vi "Module - Page Execute.vi"(11 "Stop":bool) -> ()   [LabVIEW 2020]
uses:
  Control/Setup - Sequence Data.ctl
  Control/Setup - Sequence Data Label.ctl
  Control/Page - Execute State.ctl
  <vilib>/Utility/NIReport.llb/NI_report.lvclass
  Control/Data to Execute.ctl
  Control/Transaction Info.ctl
  Control/Product Info.ctl
  Control/Acceptance Criteria Info.ctl
  Control/Execution Info.ctl
  Control/Results Info.ctl
  Control/Execute - Index of Elapse time.ctl
  Control/State - eFGV.ctl
  Control/Section.ctl
  <vilib>/Utility/miscctls.llb/LVPointDoubleTypeDef.ctl
  Control/State - FGV.ctl
  <vilib>/Utility/NIReport.llb/Report Type.ctl
  <vilib>/Utility/file.llb/Write Delimited Spreadsheet (string).vi
  <userlib>/_OpenG.lib/comparison/comparison.llb/Boolean Changed__ogtk.vi
  <vilib>/Utility/NIReport.llb/Append Report Text (str wrap).vi
  <vilib>/Utility/NIReport.llb/NI_ReportGenerationCore.lvlib
panel:
  out "SequenceNoFolder":string
  out "Test Status Ind":string
  out "Hold Time Remainder":dbl
  in  "TARE":bool caption="1"
  in  "End Mark":bool caption="1"
  in  "Test Type":string(combo)
  in  "Execute Tab":enum32{"Test", "Info", "Misc."}(tab)
  out "Holding Started":bool
  in  "Chart No":string
  out "Overall Status":bool
  in  "Table Reading":i32(listbox)
  out "% Test Completed":dbl format="%.1f %"
  out "%Pressure Stabilized":dbl caption="% Pressure Stabilized" format="%.1f %"
  out "Holding Pressure Drop (Psi)":dbl
  out "Low Pressure":bool
  in  "Pause/Resume":bool
  in  "Execute View":string="View"
  in  "Execute Reading":string="Reading"
  in  "Execute Key Value":string="Key Value" caption="Info"
  in  "Execute Info":string="Info" caption="Info"
  out "Blow Down  Test":bool
  out "Hold Time (hh:mm)":string
  out "Test Pressure":i32 format="%.0f psi"
  in  "tab - View Data":T1(tab)
  in  "Start Marker":u32(colorbox)=16860
  in  "Plot Colour":u32(colorbox)=16711680
  in  "Stop Marker":u32(colorbox)=1441830
  in  "Grid Colour":u32(colorbox)=35170
  out "Polar Plot":picture
  out "Linear Graph":cluster{"Time ,x":dbl[], "Magnitude ,y":sgl[]}(graph)
  in  "Statistic":i32(listbox)
  out "Key Value Remain Hold Time":string="00:00:00" caption="Holding Time"
  out "Key Value Recording Duration":string="00:00:00" caption="Recording Duration"
  out "Key Value Current Pressure (psi)":sgl caption="Current Pressure (psi)" format="%.1f psi"
  in  "Run Test":bool caption="1"
  out "Remain Hold Time":string="00:00:00"
  out "Holding Pressure (psi)":dbl
  out "Current Pressure (psi)":sgl format="%.1f"
  in  "Clear Mark":bool caption="1"
  in  "Start Mark":bool caption="1"
  in  "Finish":bool caption="1"
  out "Start Holding Datetime":string
  out "End Holding Datetime":string
  out "Recorded Holding Time":string
  out "Start Holding Pressure (psi)":string
  out "End Holding Pressure (psi)":string
  out "Different in Holding Pressure,psi(%)":string
  out "Permitted Holding Pressure Drop, psi%":string
  out "Recording Duration":string="00:00:00"
  in  "View":string(combo)
  out "Test Sequence":string
  out "Seq.No":string
  out "Variance":string
  out "Transaction Number":u16
  out "Test Requirement":string
  out "Test Media":string
  out "Notes":string
  out "PSL":string
  in  "Test System Description":string caption="Test System"
  out "Rework":bool caption="Rework?"
  out "Ref Order No.":dbl caption="Ref. Order No."
  out "NCR No.":string
  in  "Header multi-test 3":T2={"Seq.SelectRun 4"="Select", "Seq.Done"="Status", "Seq.No"="Run?", "Seq.No 2"="Test Sequence", "Seq.No 3"="No.", "Seq.No 4"="Test Req. ID", "Seq.No 5"="Test Requirement", "Seq.No 6"="Variance", "Seq.No 7"="Test Procedure", "Seq.No 8"="Section", "Seq.No 9"="Test Bunker", "Seq.No 10"="Test Media", "Seq.No 11"="Test Pressure (psi)", "Seq.No 12"="Cycle", "Seq.No 13"="Holding time (hh:mm)", "Seq.No 14"="Chart Scale", "Seq.No 15"="Blowdown? (y/n)", "Seq.No 16"="Actuator Pressure (psi)", "Seq.No 17"="Max. Blowdown Pressure (psi)"}
  out "Sequence List":T3[](array[typedef])
  in  "Label.Test":string="Test" caption="Test"
  out "Test Category list":string="SUT 9, Hydro"
  in  "Test System":string
  in  "Test Category":string
  out "Material Description":string caption="Material List"
  out "Material":string
  out "Project":string
  out "Customer Description":string caption="Customer List"
  in  "Test System Name":string
  in  "Procedure No./Ref.":string caption="X-Document No./Ref."
  out "Working Pressure":string
  in  "Test System":string
  out "Rev.":string
  out "Product Category":string
  out "BOM Rev.":dbl
  out "Sale Order":string caption="Sales Order"
  out "Customer":string
  out "NCR":string
  out "Order Number":string
  out "Quantity":u16=1 min=1 step=1
  out "Auto Stop Test":bool caption="Automatic Stop Test after Hold Time Countdown"
  out "Auto Set Marker":bool caption="Automatic set start marker upon pressure stabilized"
  in  "Header.Tool":T4={"Type "="Type", "Id"=" ID", "Description"="Description", "Serial No"="Serial No"} caption="Header Tool"
  out "Table.Tool":i32(listbox) caption="Detail Sensor"
  out "Table.Sensor":i32(listbox) caption="Detail Sensor"
  in  "Header.Sensor":T5={"Type "="Type", "Id"=" ID", "Description"="Description", "Serial No"="Serial No", "LP"="LP"} caption="Header Detail Sensor"
  in  "Label.Result":string="Result" caption="Result"
  out "Output Set Company":string
  out "ListBox.Output Set":string caption="Output Set"
  in  "Label.Production Order Details":string="Production Order Details" caption="Production Order Details"
  out "Indicator.Sub Operation":string caption="Sub Operation"
  out "Indicator.Confirmation No":u32 caption="Confirmation No"
  out "Indicator.Operation":string caption="Operation"
  out "Indicator.Sequence No":u16 caption="Sequence No"
  out "Indicator.Order Number":u32 caption="Order Number"
  in  "Label.Tools":string="Tools" caption="Tools"
  in  "Label.Sensor":string="Sensor" caption="Sensor"
  in  "Label.Additional Procedures No./Ref.":string="Additional Procedures No./Ref." caption="Additional Procedures No./Ref."
  out "Table.Procedure No./Ref.":i32(listbox)
  out "Acceptance Criteria":string="Acceptance Criteria"
  out "% Permitted Holding Pressure":string="% per hour (vs. start holding pressure)"
  out "% Test Pressure":string=" % on top of the test pressure"
  out "Permitted Holding Pressure Drop":dbl
  out "Max Start Holding Pressure":dbl caption="Maximum Start Of Holding Pressure"
  # "EXECUTE"
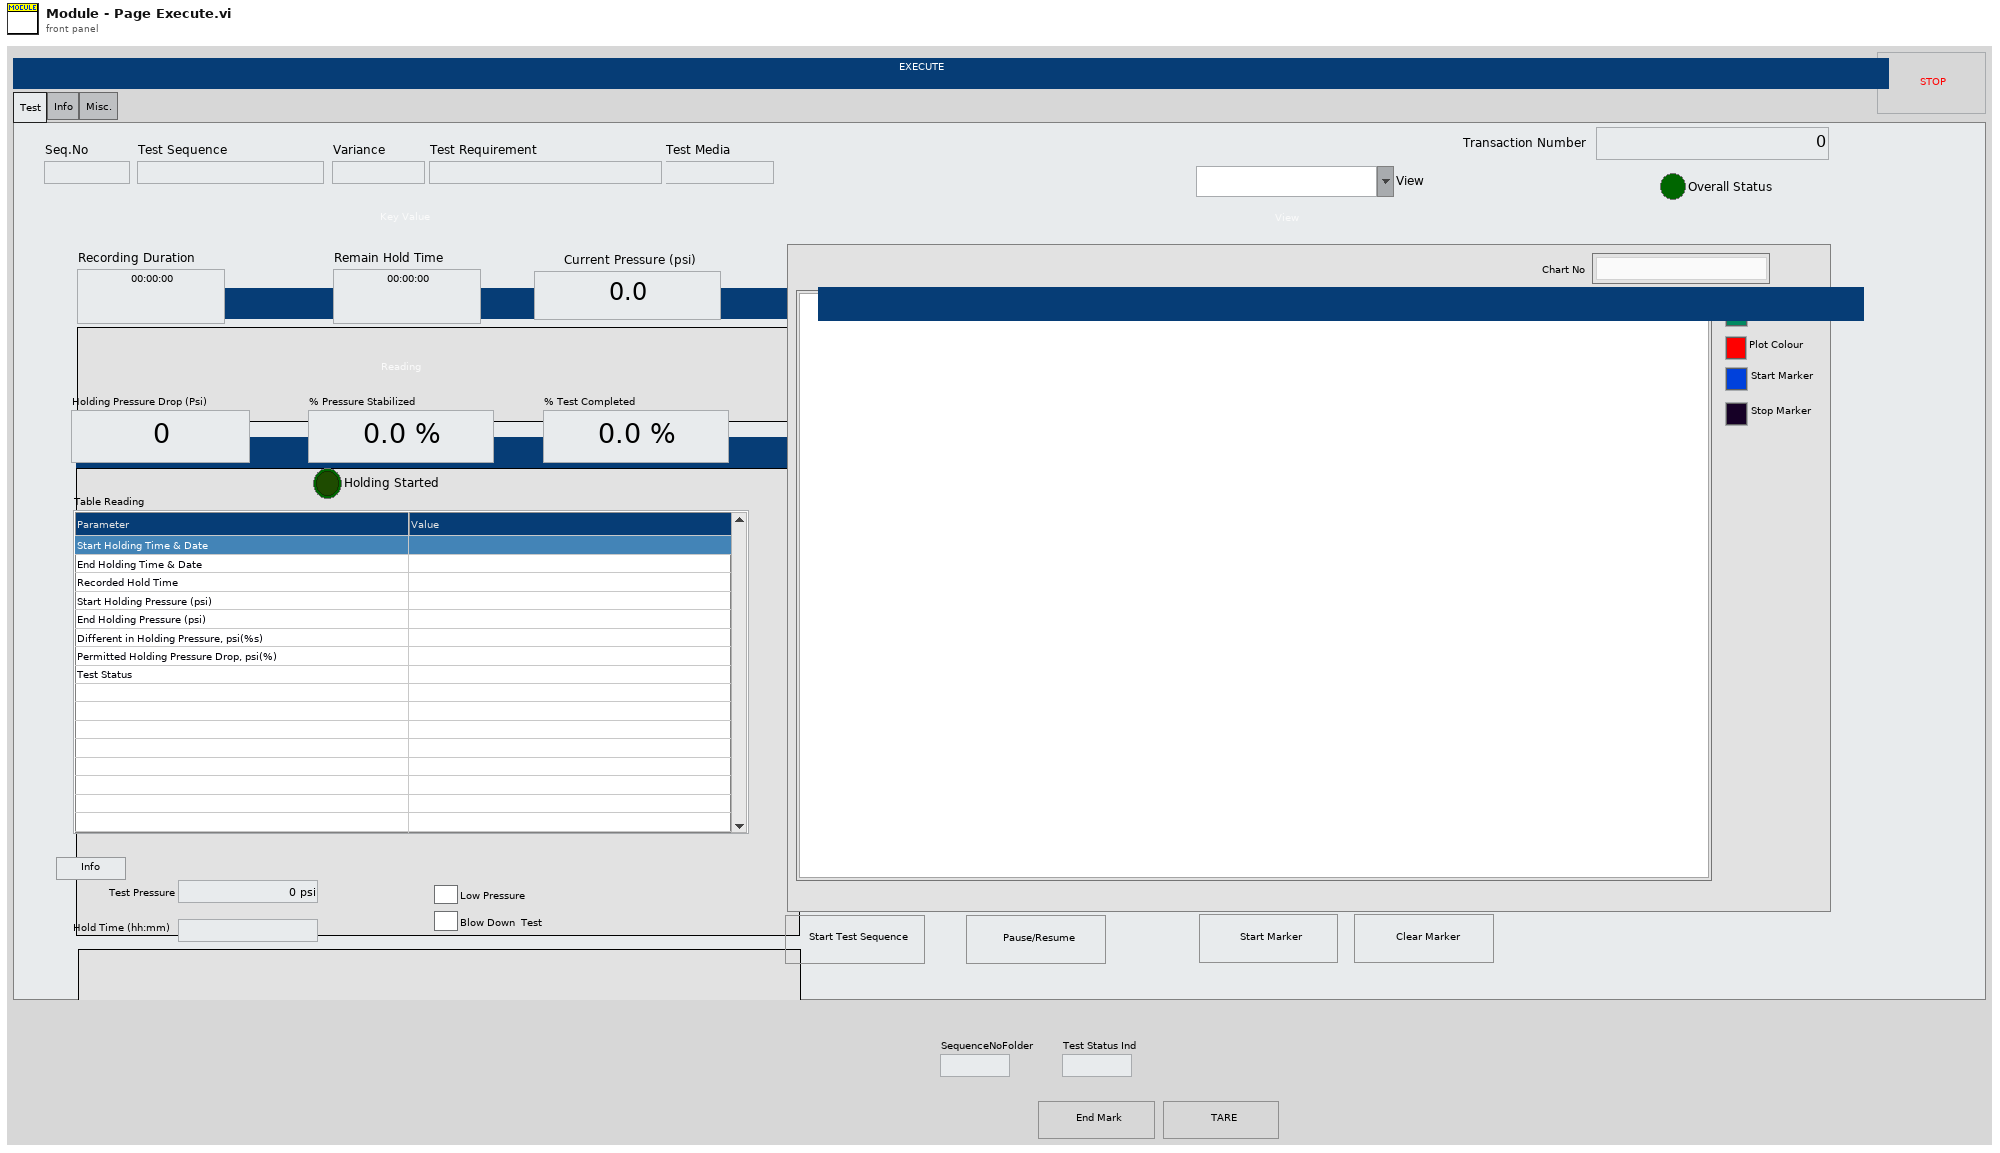
[diagram p1: front panel]
types:
  T1 = enum32{"Polar Plot", "Linear", "Statistic", "Key Value"}
  T2 = typedef "Setup - Sequence Data Label.ctl" = cluster{"Seq.SelectRun 4":string, "Seq.Done":string, "Seq.No":string, "Seq.No 2":string, "Seq.No 3":string, "Seq.No 4":string, "Seq.No 5":string, "Seq.No 6":string, "Seq.No 7":string, "Seq.No 8":string, "Seq.No 9":string, "Seq.No 10":string, "Seq.No 11":string, "Seq.No 12":string, "Seq.No 13":string, "Seq.No 14":string, "Seq.No 15":string, "Seq.No 16":string, "Seq.No 17":string}
  T3 = typedef "Setup - Sequence Data.ctl" = cluster{"Seq.Select":bool, "Seq.Status":u32, "Seq.Run":bool, "Seq.TestSequence":string, "Seq.No":string, "Seq.ReqID":string, "Seq.TestReq":string, "Seq.Variance":string, "Seq.TestProcedure":string, "Seq.Section":string, "Seq.TestBunker":string, "Seq.TestMedia":string, "Seq.TestPressure":string, "Seq.Cycle":string, "Seq.HoldingTime":string, "Seq.ChartScale":string, "Seq.BDIndicator":string, "Seq.ActuatorPressure":string, "Seq.MaxBDPressure":string}
  T4 = cluster{"Type ":string, "Id":string, "Description":string, "Serial No":string}
  T5 = cluster{"Type ":string, "Id":string, "Description":string, "Serial No":string, "LP":string}
  T6 = typedef "Execute - Index of Elapse time.ctl" = enum16{"Elapse Gap Data", "Holding Time", "Recording Duration"}
  T7 = typedef "Data to Execute.ctl" = cluster{"Transaction Info":T8, "Product Info":T9, "Misc - Additional Refs":string[][], "Misc - Sensors":string[][], "Misc - Tools":string[][], "Acceptance Criteria Info":T10, "Execution Info":T11, "Results Info":T12, "Notes":string}
  T8 = typedef "Transaction Info.ctl" = cluster{"Transaction Number":u32, "Order Number":u32, "Quantity":u16, "Customer":u32, "Customer Description":string, "Project":string, "Sales Order":u32, "Material":u32, "Material Description":string, "Rework":bool, "NCR No.":string, "Ref Order No.":dbl, "Item No.":u32, "BOM Rev.":dbl}
  T9 = typedef "Product Info.ctl" = cluster{"Product Category":string, "Procedure No./Ref.":string, "Test System":string, "Test System Description":string, "Working Pressure":string, "Pressure Unit":string, "Rev.":string, "PSL":string}
  T10 = typedef "Acceptance Criteria Info.ctl" = cluster{"Max Start Hold Pressure":dbl, "Enum.Max Start Hold Pressure":enum16{"%", "psi"}, "Permitted Hold Pressure Drop":dbl, "Enum.Permitted Hold Pressure Drop":enum16{"%", "psi"}}
  T11 = typedef "Execution Info.ctl" = cluster{"Auto Set Marker":bool, "Auto Stop Test":bool}
  T12 = typedef "Results Info.ctl" = cluster{"ListBox.Output Set":string, "Output Set Description":string}
  T13 = cluster{"T_Out":i32, "Point Phase":dbl[], "polar attributes":cluster{"maximum":dbl, "minimum":dbl, "clip to min":bool, "log?(F)":bool, "grid color":u32, "plot color":u32, "fmt and prec":cluster{"format":enum8{"Decimal", "Scientific", "Engineering", "Binary", "Octal", "Hex"}, "precision":u8}, "visible section":u16}, "Current Pressure":sgl, "Counter Time":dbl, "marking plot colour":u32, "Active Cursor":u32, "Event AI Data":sgl[], "Run Test":bool, "Config":cluster{"Holding Pressure":dbl, "Set Polar Time":dbl}, "Array of Elapse Time":timestamp[], "Remaining Holding Time":dbl, "Max Pressure":sgl, "Start Mark":bool, "Plot length (min)":dbl, "Plot length scale":dbl, "Magnitude ,y":sgl[], "Time ,x":dbl[], "Result Elapse":dbl[], "Phase":dbl[], "data array [mag, phase (deg)]":cluster{"magnitude":dbl, "phase":dbl}[], "Max Phase":dbl, "Plot and scale":cluster{"Size Linear plot":u16, "Size point plot":u16, "Plot Scale":dbl}, "Start Holding Pressure (psi)":dbl, "End Holding Pressure (psi)":dbl, "Marking Data":cluster{"magnitude 2":dbl, "phase":dbl}[], "Display Polar Scale":cluster{"Time Scale Label":string, "Max Scale label":string}, "report out":refnum<class "NI_report.lvclass">, "axis labels":string[], "Polar Picture":picture, "Event Ref":refnum<event-registration>, "Data to Execute":T7, "Sequence Data":T3[], "Holding Starter?":bool, "%Pressure Stabilized":dbl, "Target Holding Time":dbl, "Datalog path":path, "AI Offset":sgl[], "Sequence Number":i32, "Current Sequence":T3, "All Sequence Done":bool, "Sequence Started":bool}
  T14 = typedef "Page - Execute State.ctl" = enum16{"Init", "Register Event", "Read Config File", "Idle", "Start Marking", "Clear Mark", "Init Test Param", "Init File and Folder", "Get Current Sequence", "Cal Elapse Time", "Display Data", "Check Start Holding", "Polar attributes", "Insert Acc Data", "Convert Time To Phase", "Get Plot length", "Polar linear Plot", "Polar Point", "Plot linear Graph", "Update Table Data", "Display Holding Time", "Display Result Test", "Display Label", "Finish Test", "Setup Cop", "Merge Picture", "Save  Data", "Get Next Sequence", "Create Report", "Fillup Report", "Process", "Update Info - Transaction", "Update Info - Product", "Update Info - Additional Refs", "Update Info - Sensors", "Update Info - Tools", "Update Info - Acceptance Criteria", "Update Info - Execution", "Update Info - Results", "Update Info - Notes", "Close"}
  T15 = typedef "Section.ctl" = enum16{"Software Setup", "Config", "Setup", "Network Stream", "MQTT Client", "Setting", "Sample Interval", "Calibration", "Pre-Ranging", "Overrun", "Static", "Filter", "Properties", "Alarm", "Device", "Logging"}
  T16 = typedef "LVPointDoubleTypeDef.ctl" = cluster{"X":dbl, "Y":dbl}
  T17 = typedef "State - FGV.ctl" = enum16{"Write", "Read"}
  T18 = enum8{"Decimal", "Scientific", "Engineering", "Binary", "Octal", "Hex"}
  T19 = cluster{"polar attributes":cluster{"maximum":dbl, "minimum":dbl, "clip to min":bool, "log?(F)":bool, "grid color":u32, "plot color":u32, "fmt and prec":cluster{"format":enum8{"Decimal", "Scientific", "Engineering", "Binary", "Octal", "Hex"}, "precision":u8}, "visible section":u16}, "data array [mag, phase (deg)]":cluster{"magnitude":dbl, "phase":dbl}[], "font":cluster{"desired font(Application) ":enum16{"User-specified Font", "Application Font", "System Font", "Dialog Font"}, "[user-specified font] ":cluster{"Font Name:":string, "Size":i16, "Strikeout?":bool, "Italic?":bool, "Underline?":bool, "Outline?":bool, "Shadow?":bool, "Bold?":bool}}, "Scale Polar plot":dbl, "Size":u16}
  T20 = cluster{"Execute Data":string[], "Sequence no":string}
  T21 = typedef "State - eFGV.ctl" = enum16{"Init", "Read", "Write", "Exit"}
  T22 = typedef "NI_ReportGenerationCore.lvlib/Report Type.ctl" = enum16{"HTML", "Word", "Excel"}
  T23 = cluster{"position (excel)":cluster{"row":i32, "column":i32}, "name (excel)":string, "bookmark (word)":string}
  T24 = cluster{"Time Scale Label":string, "Max Scale label":string}
  T25 = cluster{"Size Linear plot":u16, "Size point plot":u16, "Plot Scale":dbl}
  T26 = cluster{"maximum":dbl, "minimum":dbl, "clip to min":bool, "log?(F)":bool, "grid color":u32, "plot color":u32, "fmt and prec":cluster{"format":enum8{"Decimal", "Scientific", "Engineering", "Binary", "Octal", "Hex"}, "precision":u8}, "visible section":u16}
  T27 = typedef "LVBoundsTypeDef.ctl" = cluster{"Width":u32, "Height":u32}
  T28 = typedef "imagedata.ctl" = cluster{"image type":i32, "image depth":i32, "image":u8[], "mask":u8[], "colors":u32[], "Rectangle":cluster{"left":i16, "top":i16, "right":i16, "bottom":i16}}
  T29 = enum32{"invalid app kind", "Development System", "Run Time System", "Student Edition", "Embedded LabVIEW", "Evaluation", "Custom"}
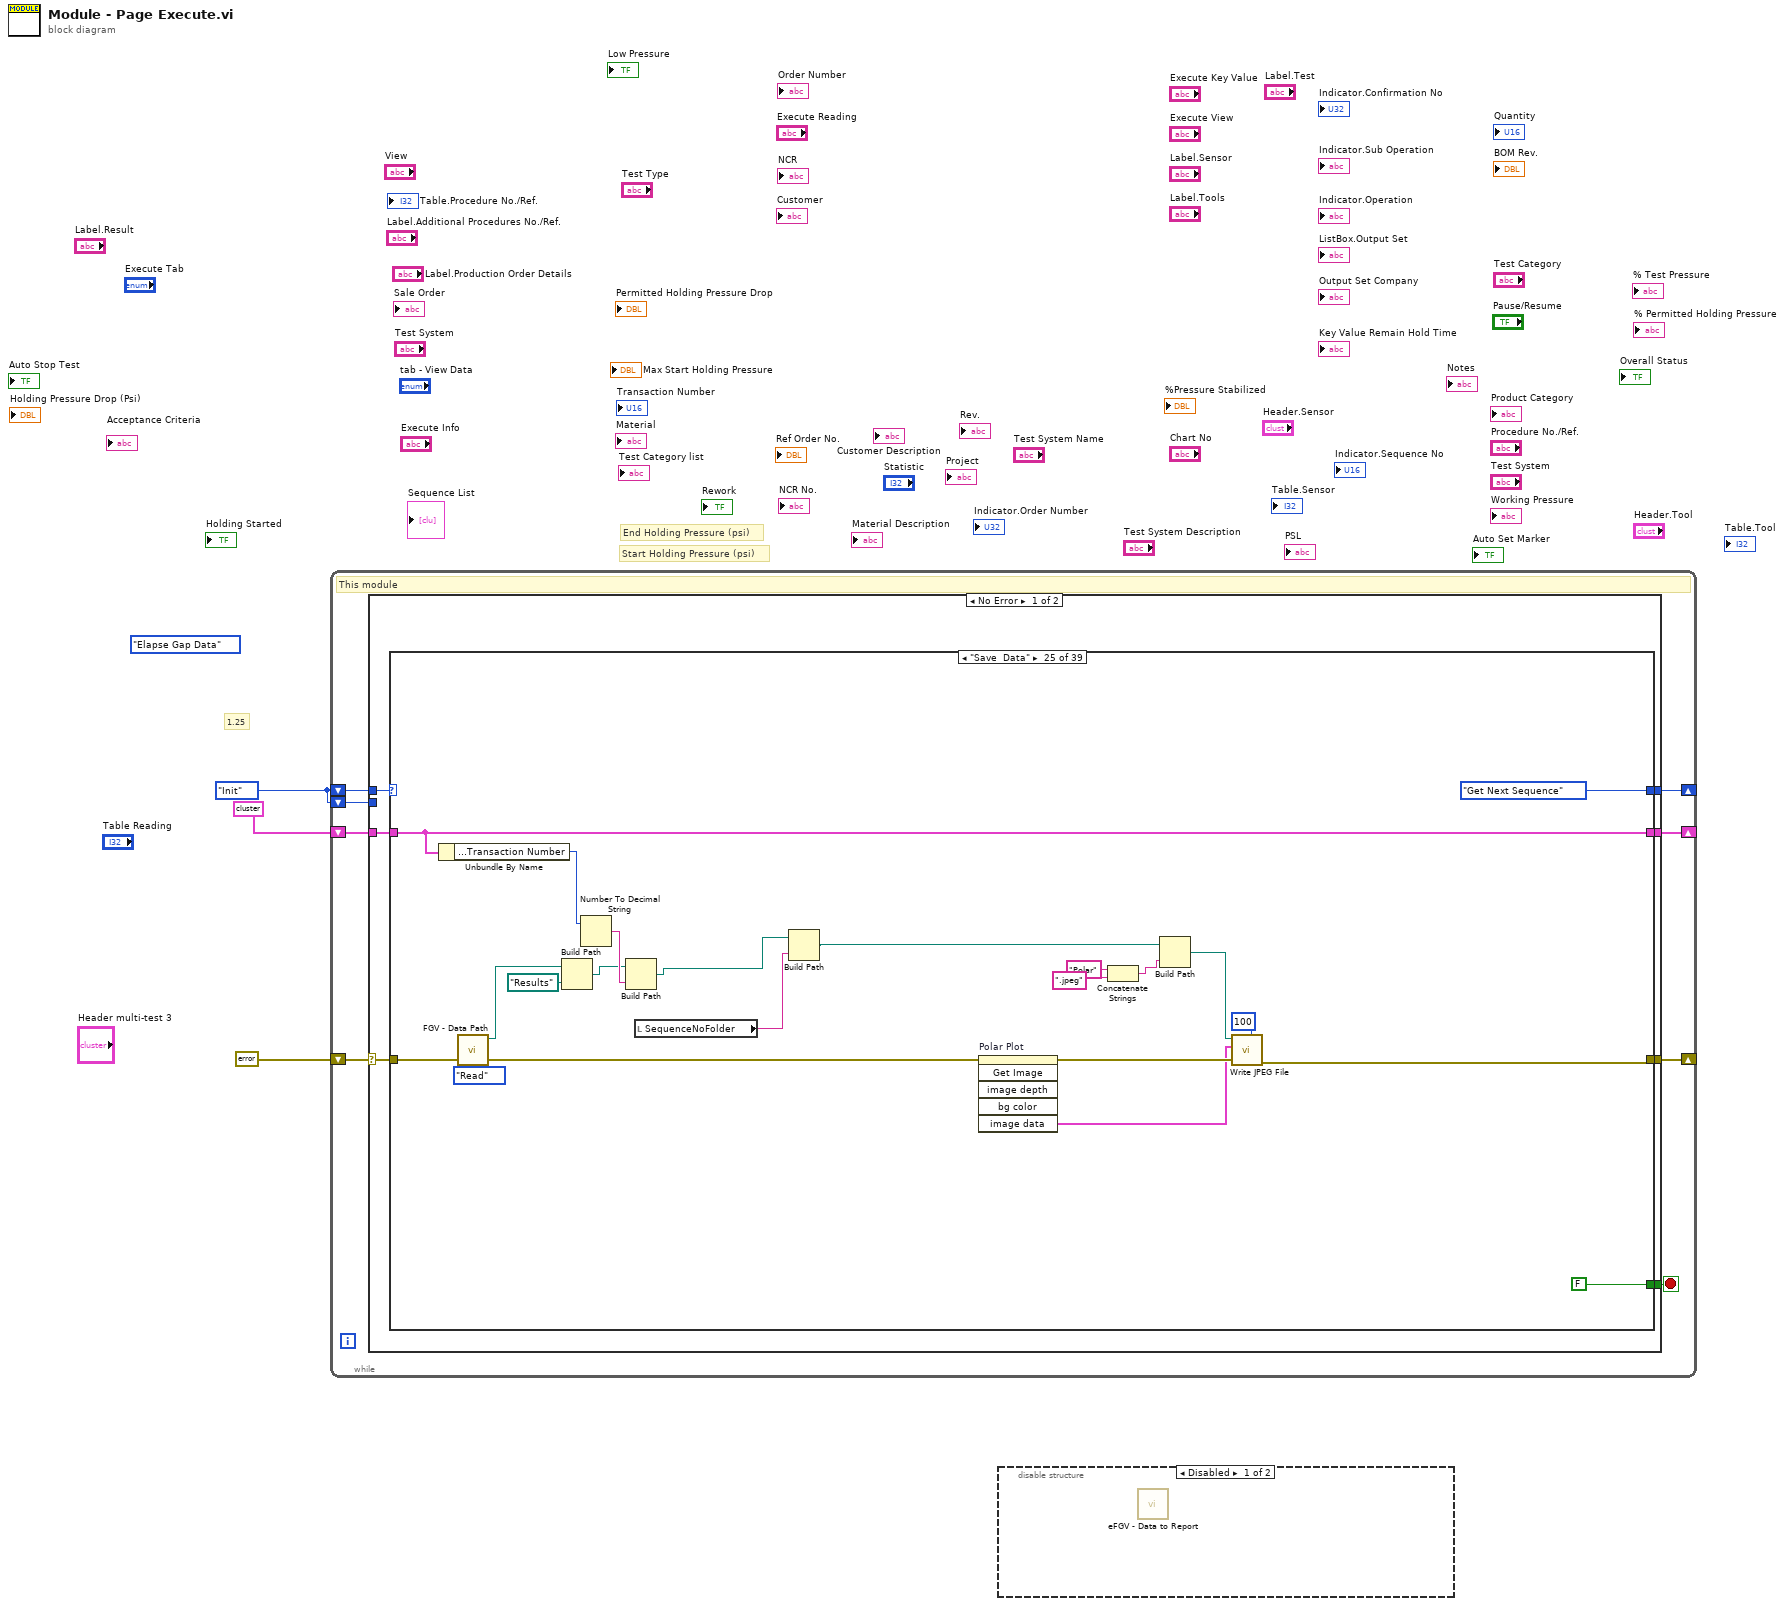
[diagram p0: block diagram]
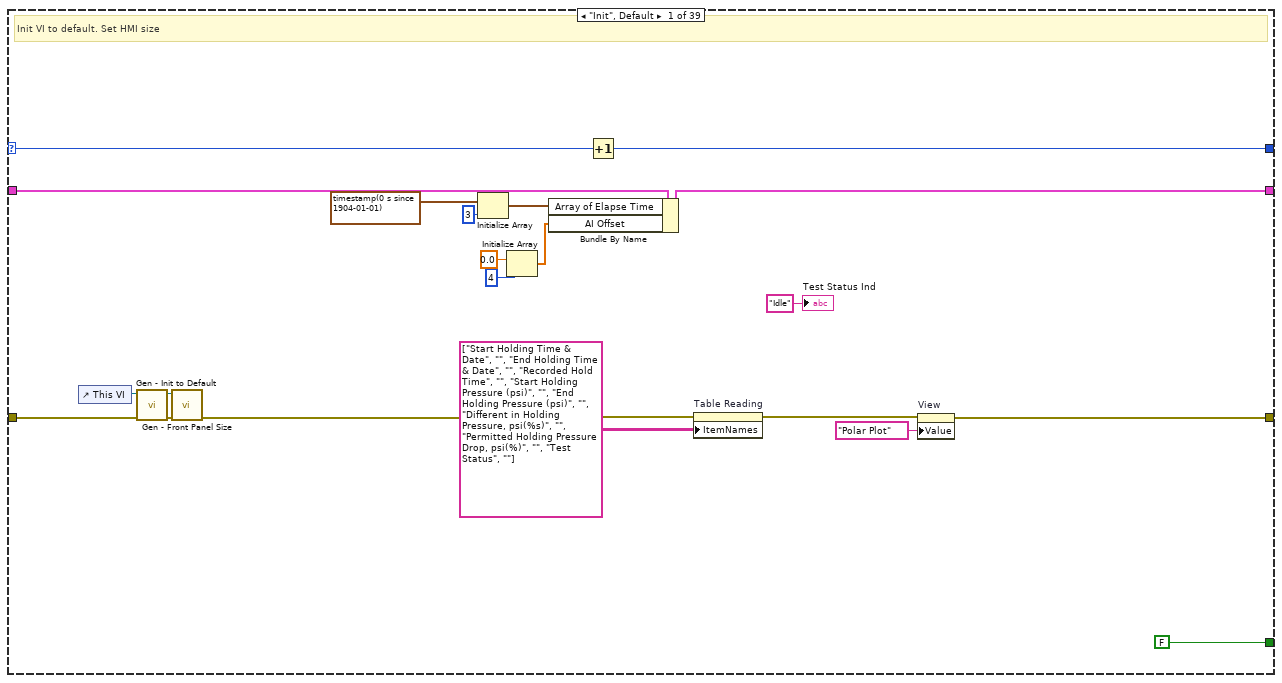
[diagram p3: hidden frame]
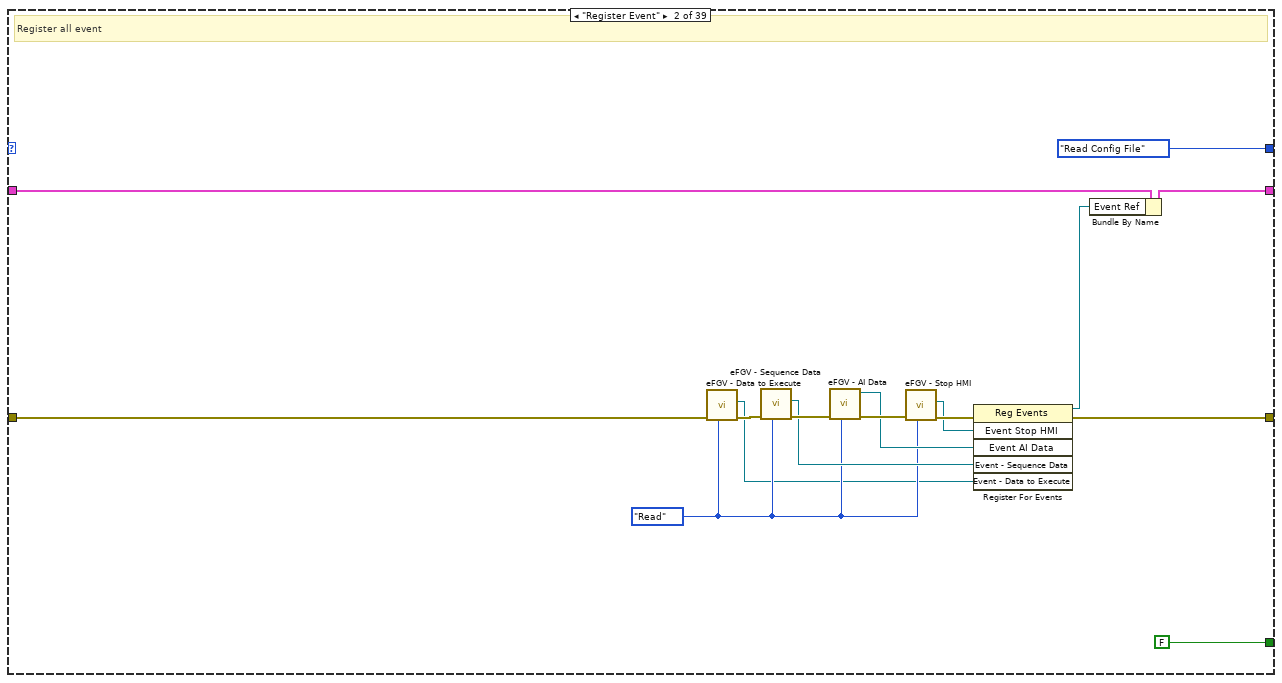
[diagram p4: hidden frame]
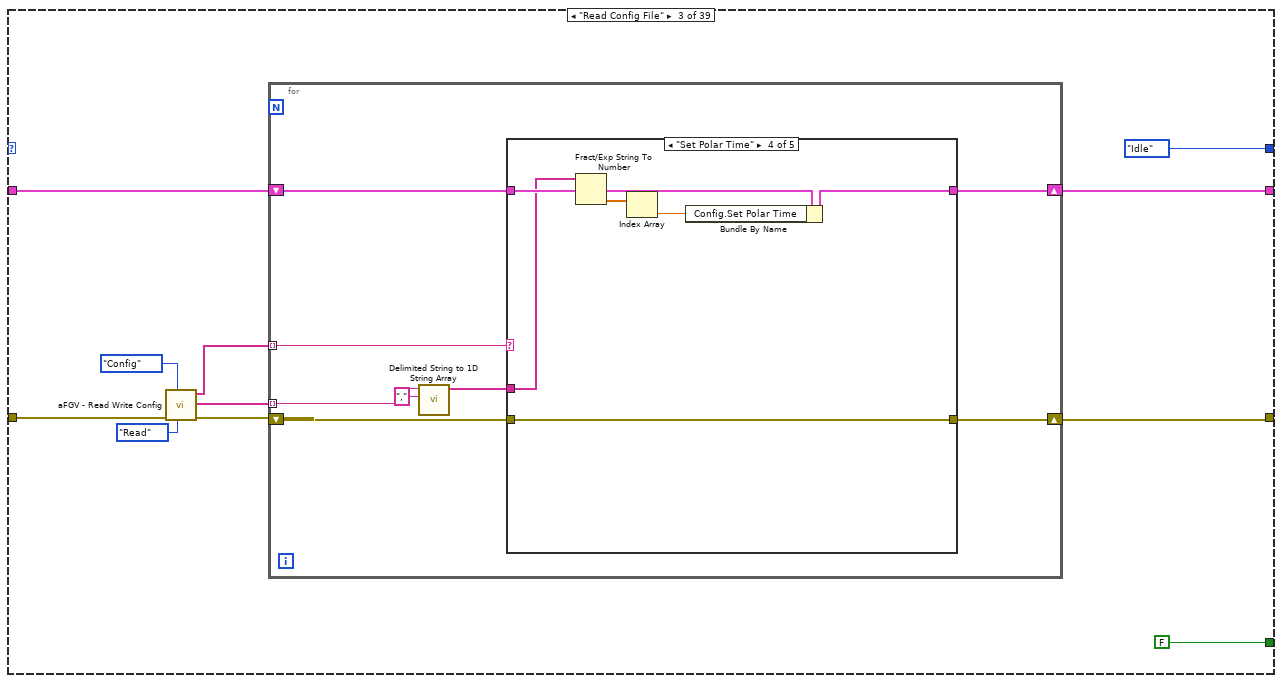
[diagram p5: hidden frame]
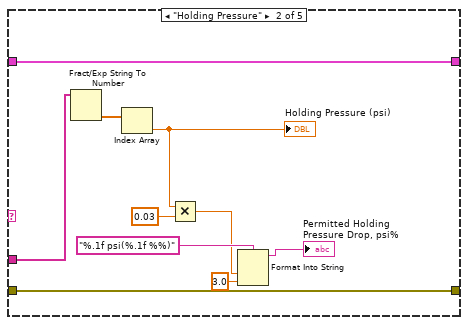
[diagram p7: hidden frame]
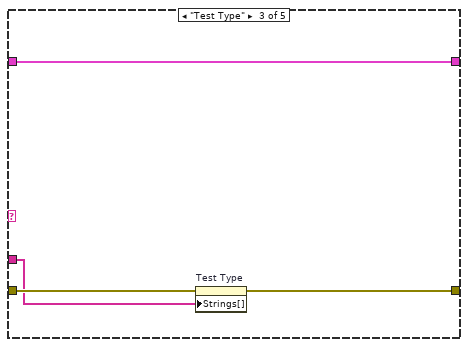
[diagram p8: hidden frame]
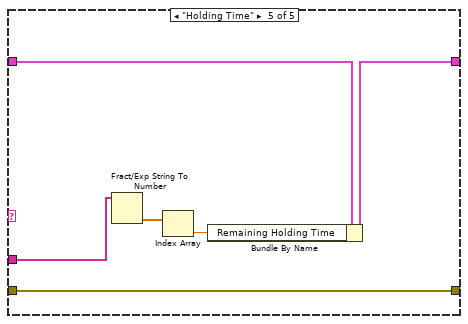
[diagram p9: hidden frame]
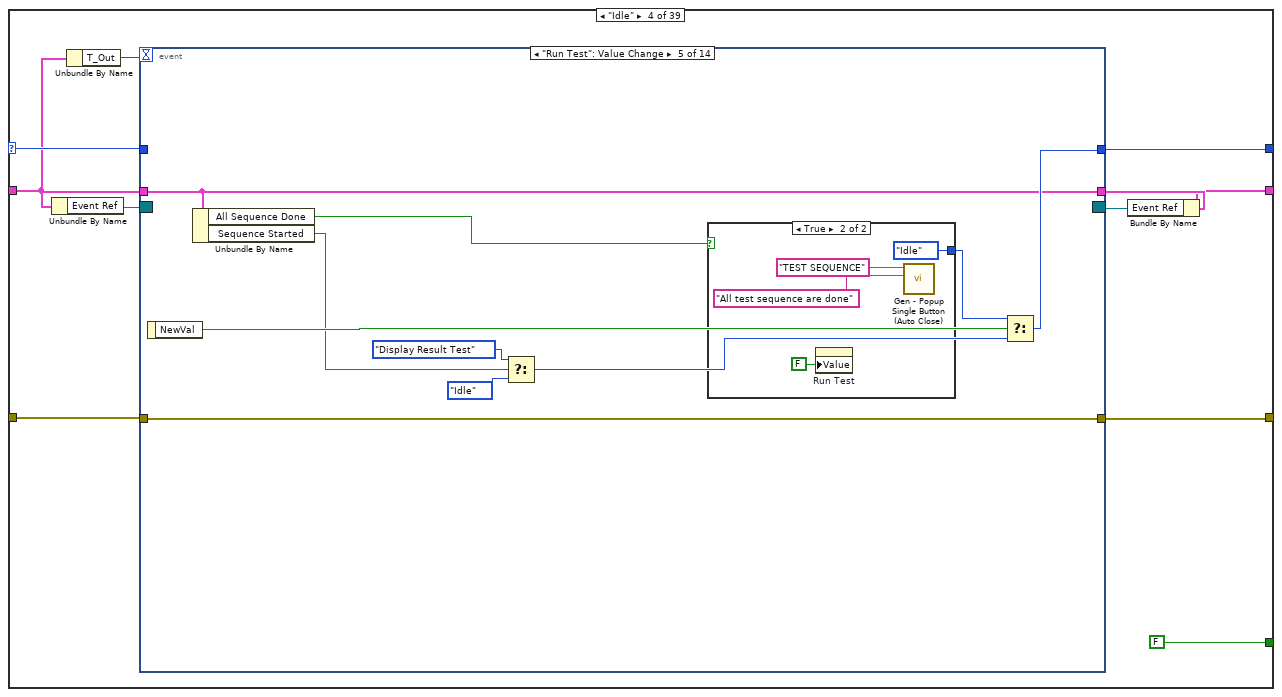
[diagram p10: hidden frame]
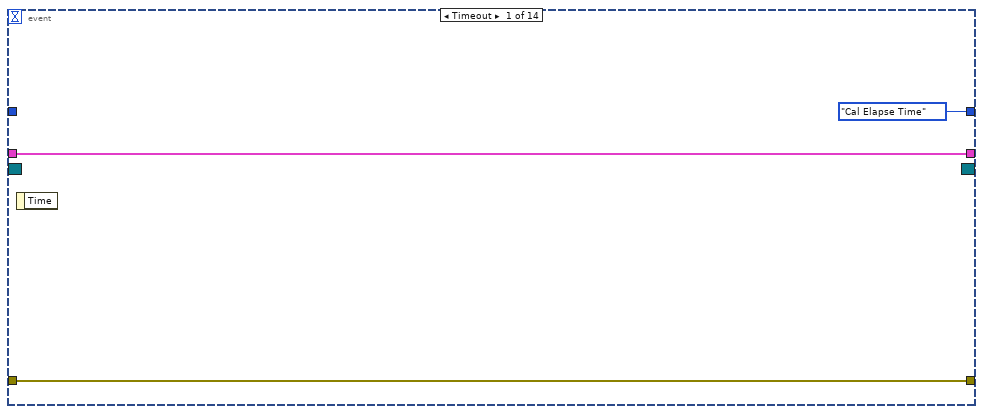
[diagram p11: hidden frame]
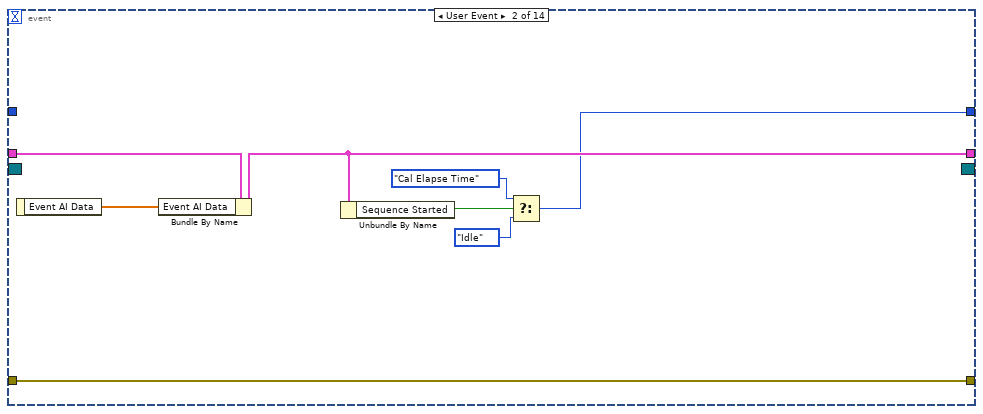
[diagram p12: hidden frame]
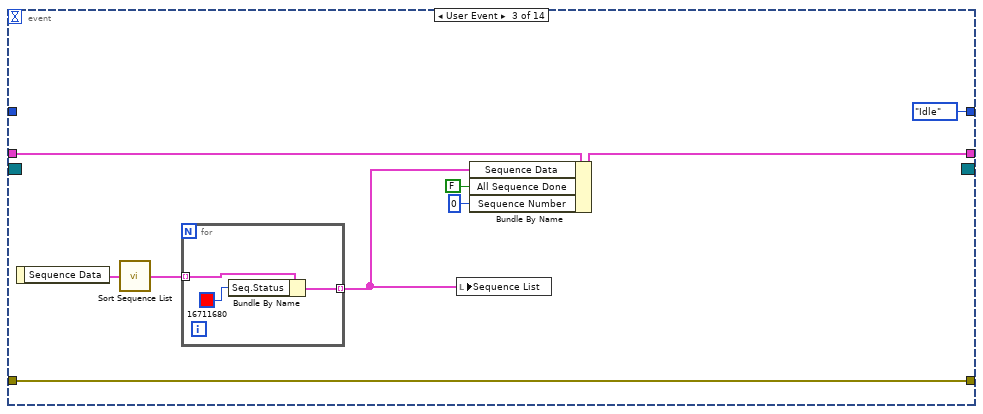
[diagram p13: hidden frame]
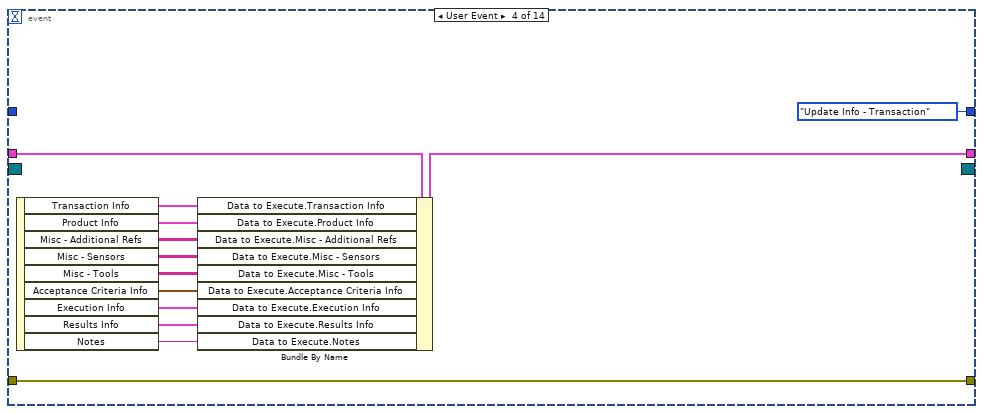
[diagram p14: hidden frame]
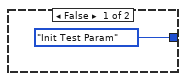
[diagram p15: hidden frame]
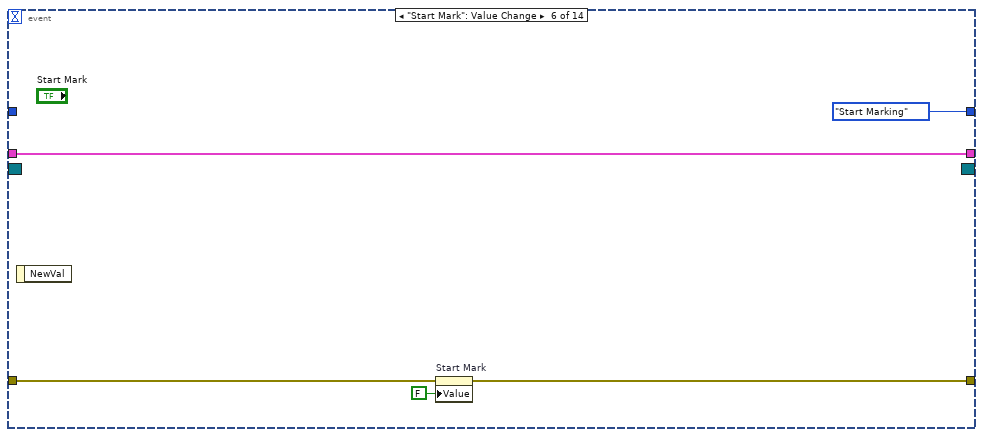
[diagram p16: hidden frame]
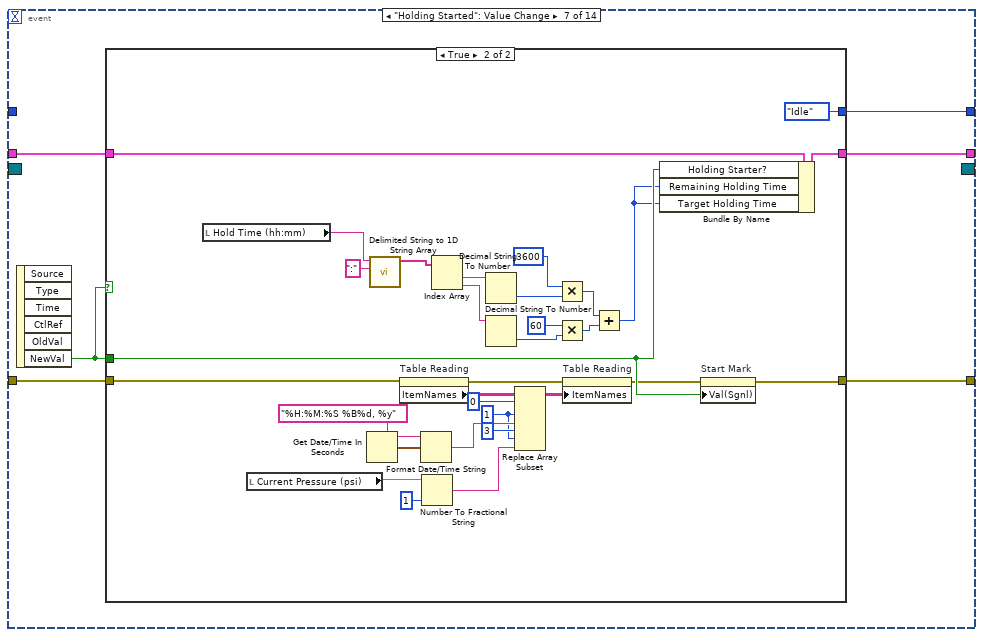
[diagram p17: hidden frame]
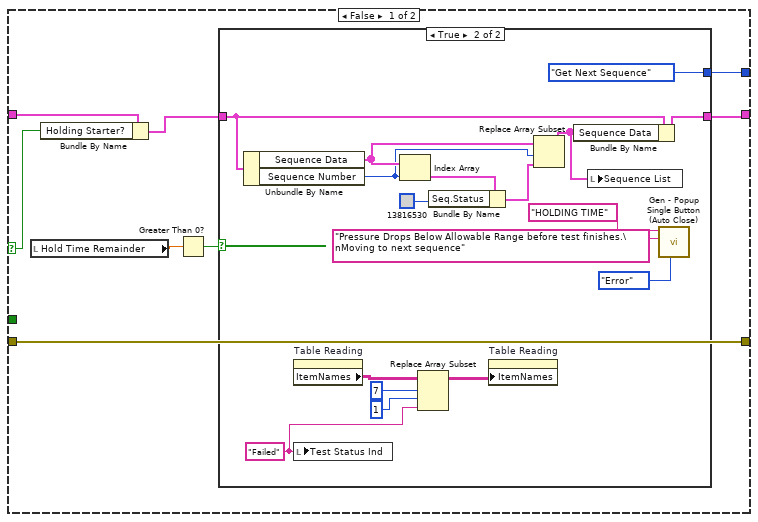
[diagram p18: hidden frame]
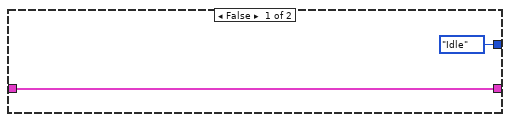
[diagram p19: hidden frame]
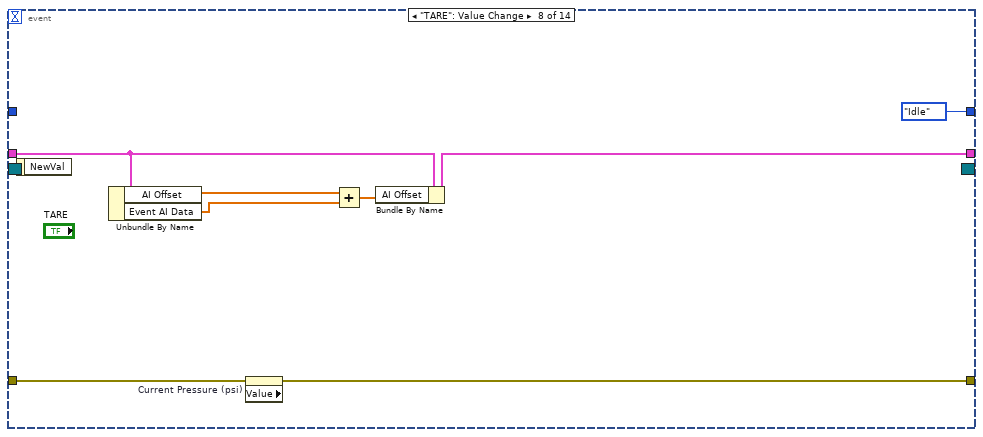
[diagram p20: hidden frame]
diagram:
  (unwired) Execute_-_Index_of_Elapse_time."Elapse Gap Data"
  w2 = Page_-_Execute_State."Init"
  # "Start Holding Pressure (psi)"
  # "End Holding Pressure (psi)"
  # "1.25"
  n1 = while {
    shift-right: [w7] -> _
    shift-left: w2 -> [w9]
    shift-right: [w10] -> _
    shift-left: errorcluster {"status"=FALSE, "code"=0, "source"=""} ("Error In") -> [w11]
    shift-right: [w5] -> _
    shift-left: T13 {"T_Out"=-1, "Point Phase"=[], "polar attributes"={"maximum"=0.0, "minimum"=0.0, "clip to min"=FALSE, "log?(F)"=FALSE, "grid color"=6710886, "plot color"=16711680, "fmt and prec"={"format"=enum."Decimal", "precision"=0}, "visible section"=8}, "Current Pressure"=0.0, "Counter Time"=0.0, "marking plot colour"=0, "Active Cursor"=0, "Event AI Data"=[], "Run Test"=FALSE, "Config"={"Holding Pressure"=0.0, "Set Polar Time"=0.0}, "Array of Elapse Time"=[], "Remaining Holding Time"=0.0, "Max Pressure"=0.0, "Start Mark"=FALSE, "Plot length (min)"=2.0, "Plot length scale"=3.0, "Magnitude ,y"=[], "Time ,x"=[], "Result Elapse"=[], "Phase"=[], "data array [mag, phase (deg)]"=[], "Max Phase"=0.0, "Plot and scale"={"Size Linear plot"=3, "Size point plot"=6, "Plot Scale"=0.2}, "Start Holding Pressure (psi)"=0.0, "End Holding Pressure (psi)"=0.0, "Marking Data"=[], "Display Polar Scale"={"Time Scale Label"="", "Max Scale label"=""}, "report out"=refnum, "axis labels"=["", "90", "180", "270"], "Polar Picture"=bytes[4090], "Event Ref"=refnum, "Data to Execute"={"Transaction Info"={"Transaction Number"=0, "Order Number"=0, "Quantity"=0, "Customer"=0, "Customer Description"="", "Project"="", "Sales Order"=0, "Material"=0, "Material Description"="", "Rework"=FALSE, "NCR No."="", "Ref Order No."=0.0, "Item No."=0, "BOM Rev."=0.0}, "Product Info"={"Product Category"="", "Procedure No./Ref."="", "Test System"="", "Test System Description"="", "Working Pressure"="", "Pressure Unit"="", "Rev."="", "PSL"=""}, "Misc - Additional Refs"=[], "Misc - Sensors"=[], "Misc - Tools"=[], "Acceptance Criteria Info"={"Max Start Hold Pressure"=0.0, "Enum.Max Start Hold Pressure"=enum."%", "Permitted Hold Pressure Drop"=0.0, "Enum.Permitted Hold Pressure Drop"=enum."%"}, "Execution Info"={"Auto Set Marker"=FALSE, "Auto Stop Test"=FALSE}, "Results Info"={"ListBox.Output Set"="", "Output Set Description"=""}, "Notes"=""}, "Sequence Data"=[], "Holding Starter?"=FALSE, "%Pressure Stabilized"=0.0, "Target Holding Time"=0.0, "Datalog path"=path "", "AI Offset"=[], "Sequence Number"=0, "Current Sequence"={"Seq.Select"=FALSE, "Seq.Status"=0, "Seq.Run"=FALSE, "Seq.TestSequence"="", "Seq.No"="", "Seq.ReqID"="", "Seq.TestReq"="", "Seq.Variance"="", "Seq.TestProcedure"="", "Seq.Section"="", "Seq.TestBunker"="", "Seq.TestMedia"="", "Seq.TestPressure"="", "Seq.Cycle"="", "Seq.HoldingTime"="", "Seq.ChartScale"="", "Seq.BDIndicator"="", "Seq.ActuatorPressure"="", "Seq.MaxBDPressure"=""}, "All Sequence Done"=TRUE, "Sequence Started"=FALSE} -> [w6]
    shift-left: w2 -> [w4]
    stop <- w8 stop-if-true
    # "This module"
    n2 = case shown="No Error" w11 {
      selector: w11 -> [w17 w966]
      tunnel: w9 -> [w16 w971]
      tunnel: [w18 w967] -> w10
      tunnel: [w15 FALSE] -> w8
      tunnel: [w14 w971] -> w7
      tunnel: w6 -> [w13 w970]
      tunnel: [w12 w970] -> w5
      tunnel: w4 -> [_ w963]
      frame No Error {
        n3 = case shown="\"Save  Data\"" w16 {
          selector: w16 -> [w33 _ _ w108 _ _ _ _ _ _ _ _ _ _ _ _ _ _ _ _ _ _ _ _ _ _ _ _ _ _ _ _ _ _ _ _ _ _ w960]
          tunnel: [w31 w55 w60 w113 w297 w319 w365 w407 w421 w472 w489 w519 w541 w562 w585 w601 w624 w663 w695 w715 w716 w738 w789 w803 w834 w849 w866 w873 w883 w904 w914 w917 w922 w927 w942 w947 w952 w956 w961] -> w18
          tunnel: w17 -> [w39 w43 w65 w112 w298 w320 w363 w419 w422 w472 w501 w520 w541 w562 w586 w602 w629 w674 w695 w715 w716 w740 w791 w804 w835 w849 w867 w878 w883 w904 w914 w918 w923 w928 w942 w947 w952 w956 w962]
          tunnel: [FALSE FALSE FALSE FALSE FALSE FALSE FALSE _ _ FALSE FALSE _ FALSE FALSE FALSE FALSE FALSE FALSE FALSE FALSE _ FALSE FALSE FALSE FALSE _ FALSE FALSE _ _ _ _ _ _ _ _ _ _ TRUE] -> w15
          tunnel: [w32 Page_-_Execute_State."Read Config File" Page_-_Execute_State."Idle" w110 Page_-_Execute_State."Idle" w315 Page_-_Execute_State."Init File and Folder" Page_-_Execute_State."Idle" Page_-_Execute_State."Idle" Page_-_Execute_State."Display Data" Page_-_Execute_State."Check Start Holding" w527 Page_-_Execute_State."Insert Acc Data" Page_-_Execute_State."Convert Time To Phase" Page_-_Execute_State."Get Plot length" Page_-_Execute_State."Polar linear Plot" Page_-_Execute_State."Polar Point" Page_-_Execute_State."Display Label" Page_-_Execute_State."Plot linear Graph" w697 Page_-_Execute_State."Display Holding Time" w729 Page_-_Execute_State."Finish Test" Page_-_Execute_State."Save  Data" Page_-_Execute_State."Get Next Sequence" w847 Page_-_Execute_State."Fillup Report" Page_-_Execute_State."Idle" Page_-_Execute_State."Idle" Page_-_Execute_State."Update Info - Product" Page_-_Execute_State."Update Info - Additional Refs" Page_-_Execute_State."Update Info - Sensors" Page_-_Execute_State."Update Info - Tools" Page_-_Execute_State."Update Info - Acceptance Criteria" Page_-_Execute_State."Update Info - Execution" Page_-_Execute_State."Update Info - Results" Page_-_Execute_State."Update Info - Notes" Page_-_Execute_State."Get Current Sequence" w960] -> w14
          tunnel: w13 -> [w37 w51 w57 w104 w295 w317 w367 w417 w447 w462 w488 w525 w544 w575 w590 w616 w631 w661 w681 w703 w718 w735 w780 w811 w825 w848 w870 w877 w882 w902 w913 w919 w924 w929 w941 w946 w951 w954 w958]
          tunnel: [w29 w50 w56 w106 w294 w318 w366 w399 w434 w470 w496 w525 w554 w568 w587 w612 w622 w659 w681 w709 w718 w734 w780 w810 w825 w846 w865 w877 w882 w902 w913 w919 w924 w929 w941 w946 w951 w954 w958] -> w12
          frame "Init", Default {
            # "Init VI to default. Set HMI size"
            n4 = control-ref of="This VI"() -> (w35:refnum<vi>)
            n5 = call "Gen - Init to Default.vi"("Error in"=w39, "This VI"=w35) -> ("Error out"=w38:errorcluster, "This VI Copy"=w34:refnum<vi>)  [unwired: 8 in]
            n6 = call "Gen - Front Panel Size.vi"("Error In"=w38, "This VI"=w34) -> ("Error Out"=w22:errorcluster)  [unwired: 9 in]
            n7 = Initialize Array(timestamp(0 s since 1904-01-01), 3 ("dimension size")) -> (w26:timestamp[])
            n8 = Initialize Array(0.0 ("element"), 4 ("dimension size")) -> (w23:dbl[])
            n9 = Bundle By Name(cluster=w37, "Array of Elapse Time"=w26, "AI Offset"=w23) -> (w29:T13)
            n10 = Increment(x=w33) -> (x+1=w32:T14)
            n11 = property on="Table Reading" class="MCListbox (strict)"(error in=w22, "ItemNames"=string[][] [["Start Holding Time & Date", ""], ["End Holding Time & Date", ""], ["Recorded Hold Time", ""], ["Start Holding Pressure (psi)", ""], ["End Holding Pressure (psi)", ""], ["Different in Holding Pressure, psi(%s)", ""], ["Permitted Holding Pressure Drop, psi(%)", ""], ["Test Status", ""]] ("Item Names")) -> (error out=w21:errorcluster)  [unwired: 1 in, 1 out]
            n12 = property on="View" class="CmbBox"(error in=w21, "Value"="Polar Plot" ("View")) -> (error out=w31:errorcluster)  [unwired: 1 in, 1 out]
            "Test Status Ind" <- "Idle" ("Test Status Ind")
          }
          frame "Register Event" {
            w42 = State_-_eFGV."Read" ("Action")
            # "Register all event"
            n13 = call "eFGV - Data to Execute.vi"("Action"=w42, "Error In"=w43) -> ("Error Out"=w44:errorcluster, "Event - Data to Execute"=w41:refnum<user-event>)  [unwired: 8 in]
            n14 = call "eFGV - Sequence Data.vi"("States"=w42, "Error In"=w44) -> ("Error Out"=w46:errorcluster, "Event - Sequence Data"=w45:refnum<user-event>)  [unwired: 7 in, 1 out]
            n15 = call "eFGV - AI Data.vi"("States"=w42, "Error In"=w46) -> ("Error Out"=w48:errorcluster, "Event AI Data"=w47:refnum<user-event>)  [unwired: 8 in]
            n16 = call "eFGV - Stop HMI.vi"("Action"=w42, "Error In"=w48) -> ("Error Out"=w54:errorcluster, "Event Stop HMI"=w52:refnum<user-event>)  [unwired: 7 in, 1 out]
            n17 = register-events(error in=w54, w52, w47, w45, w41) -> (reference out=w40:refnum<event-registration>, error out=w55:errorcluster)  [unwired: 1 in]
            n18 = Bundle By Name(cluster=w51, "Event Ref"=w40) -> (w50:T13)
          }
          frame "Read Config File" {
            n19 = call "aFGV - Read Write Config.vi"("State"=enum16{"Read", "Write", "Delete"}."Read", "Section"=Section."Config", "Error In"=w65) -> ("Error Out"=w61:errorcluster, "Data out"=w59:string[], "Key Names"=w58:string[])  [unwired: 6 in]
            n20 = for {
              shift-right: [w74] -> w60
              shift-left: w61 -> [w72]
              tunnel: w58 -> [w73] mode=indexing
              tunnel: w59 -> [w71] mode=indexing
              shift-right: [w68] -> w56
              shift-left: w57 -> [w69]
              n21 = call <vilib>:"Delimited String to 1D String Array.vi"("delimiter"=",", "delimited string"=w71) -> ("string array"=w70:string[])  [unwired: 9 in]
              n22 = case shown="\"Set Polar Time\"" w73 {
                tunnel: w72 -> [w76 w86 w89 w96 w102]
                tunnel: [w76 w86 w88 w96 w102] -> w74
                tunnel: w70 -> [_ w83 w87 w92 w99]
                tunnel: w69 -> [w75 w85 w90 w95 w101]
                tunnel: [w75 w85 w90 w94 w98] -> w68
                frame Default {
                }
                frame "Holding Pressure" {
                  n23 = Fract/Exp String To Number(string=w83) -> (number=w84:dbl[])  [unwired: 3 in, 1 out]
                  n24 = Index Array(array=w84) -> (element=w77:dbl)  [unwired: 1 in]
                  "Holding Pressure (psi)" <- w77
                  n25 = Multiply(x=w77, y=0.03) -> (x*y=w80:dbl)
                  n26 = Format Into String(format string="%.1f psi(%.1f %%)", w80, 3.0 ("input 2")) -> (resulting string=→"Permitted Holding Pressure Drop, psi%":string)  [unwired: 2 in, 1 out]
                }
                frame "Test Type" {
                  n27 = property on="Test Type" class="CmbBox"(error in=w89, "Strings[]"=w87) -> (error out=w88:errorcluster)  [unwired: 1 in, 1 out]
                }
                frame "Set Polar Time" {
                  n28 = Fract/Exp String To Number(string=w92) -> (number=w93:dbl[])  [unwired: 3 in, 1 out]
                  n29 = Index Array(array=w93) -> (element=w91:dbl)  [unwired: 1 in]
                  n30 = Bundle By Name(cluster=w95, "Config.Set Polar Time"=w91) -> (w94:T13)
                }
                frame "Holding Time" {
                  n31 = Fract/Exp String To Number(string=w99) -> (number=w100:dbl[])  [unwired: 3 in, 1 out]
                  n32 = Index Array(array=w100) -> (element=w97:dbl)  [unwired: 1 in]
                  n33 = Bundle By Name(cluster=w101, "Remaining Holding Time"=w97) -> (w98:T13)
                }
              }
            }
          }
          frame "Idle" {
            n34 = Unbundle By Name(w104) -> ("Event Ref"=w107:refnum<event-registration>)
            n35 = Unbundle By Name(w104) -> ("T_Out"=w103:i32)
            n36 = event shown="[4] \"Run Test\": Value Change" {
              selector: w107 -> [_ _ _ _ _ _ _ _ _ _ _ _ _ _]
              dyn-events: [_ _ _ _ _ _ _ _ _ _ _ _ _ _] -> w105
              timeout: w103 -> [_ _ _ _ _ _ _ _ _ _ _ _ _ _]
              tunnel: [w116 w124 w132 w149 w159 w166 w173 w240 w249 w260 w272 w287 w290 w293] -> w113
              tunnel: w112 -> [w116 w124 w132 w149 w159 w167 w174 w241 w250 w261 w275 w287 w290 w293]
              tunnel: [Page_-_Execute_State."Cal Elapse Time" w117 Page_-_Execute_State."Idle" Page_-_Execute_State."Update Info - Transaction" w157 Page_-_Execute_State."Start Marking" w170 Page_-_Execute_State."Idle" Page_-_Execute_State."Idle" Page_-_Execute_State."Clear Mark" Page_-_Execute_State."Idle" Page_-_Execute_State."Finish Test" w288 Page_-_Execute_State."Close"] -> w110
              tunnel: [w114 w121 w130 w147 w156 w169 w172 w237 w252 w264 w276 w286 w289 w292] -> w109
              tunnel: w104 -> [w114 w123 w133 w148 w156 w169 w175 w239 w254 w266 w276 w286 w289 w292]
              tunnel: w108 -> [_ _ _ _ _ _ _ _ _ _ _ _ w288 _]
              event Timeout {
                n37 = event-data() -> ()  [unwired: 1 in, 1 out]
              }
              event User Event {
                n38 = event-data() -> ("Event AI Data"=w122:sgl[])  [unwired: 1 in]
                n39 = Bundle By Name(cluster=w123, "Event AI Data"=w122) -> (w121:T13)
                n40 = Unbundle By Name(w121) -> ("Sequence Started"=w120:bool)
                n41 = Select(t=Page_-_Execute_State."Cal Elapse Time", s=w120, f=Page_-_Execute_State."Idle") -> (s? t:f=w117:T14)
              }
              event User Event {
                n42 = event-data() -> ("Sequence Data"=w129:T3[])  [unwired: 1 in]
                n43 = call "Sort Sequence List.vi"("Sequence Data In"=w129) -> ("Sequence Data Out"=w128:T3[])
                n44 = for {
                  tunnel: w128 -> [w136] mode=indexing
                  tunnel: [w134] -> w127 mode=indexing
                  n45 = Bundle By Name(cluster=w136, "Seq.Status"=u32 16711680) -> (w134:T3)
                }
                n46 = local write "Sequence List"(w127) -> ()
                n47 = Bundle By Name(cluster=w133, "Sequence Data"=w127, "All Sequence Done"=FALSE, "Sequence Number"=0) -> (w130:T13)
              }
              event User Event {
                n48 = event-data() -> ("Transaction Info"=w146:T8, "Product Info"=w145:T9, "Misc - Additional Refs"=w144:string[][], "Misc - Sensors"=w143:string[][], "Misc - Tools"=w142:string[][], "Acceptance Criteria Info"=w141:T10, "Execution Info"=w140:T11, "Results Info"=w139:T12, "Notes"=w138:string)  [unwired: 1 in]
                n49 = Bundle By Name(cluster=w148, "Data to Execute.Transaction Info"=w146, "Data to Execute.Product Info"=w145, "Data to Execute.Misc - Additional Refs"=w144, "Data to Execute.Misc - Sensors"=w143, "Data to Execute.Misc - Tools"=w142, "Data to Execute.Acceptance Criteria Info"=w141, "Data to Execute.Execution Info"=w140, "Data to Execute.Results Info"=w139, "Data to Execute.Notes"=w138) -> (w147:T13)
              }
              event "Run Test": Value Change {
                n50 = event-data() -> ("NewVal"=w158:bool)  [unwired: 1 in]
                n51 = Unbundle By Name(w156) -> ("All Sequence Done"=w154:bool, "Sequence Started"=w150:bool)
                n52 = Select(t=Page_-_Execute_State."Display Result Test" ("f"), s=w150, f=Page_-_Execute_State."Idle") -> (s? t:f=w151:T14)
                n53 = case shown="True" w154 {
                  tunnel: [Page_-_Execute_State."Init Test Param" Page_-_Execute_State."Idle"] -> w155
                  frame False {
                  }
                  frame True {
                    n54 = property on="Run Test" class="Bool (strict)"("Value"=FALSE ("Run Test")) -> ()  [unwired: 2 in, 2 out]
                    n55 = call "Gen - Popup Single Button (Auto Close).vi"("Message in"="All test sequence are done", "Header"="TEST SEQUENCE") -> ()  [unwired: 8 in, 2 out]
                  }
                }
                n56 = Select(t=w155, s=w158, f=w151) -> (s? t:f=w157:T14)
              }
              event "Start Mark": Value Change {
                n57 = event-data() -> ()  [unwired: 1 in, 1 out]
                n58 = property on="Start Mark" class="Bool (strict)"(error in=w167, "Value"=FALSE ("Start Mark")) -> (error out=w166:errorcluster)  [unwired: 1 in, 1 out]
              }
              event "Holding Started": Value Change {
                n59 = event-data() -> ("NewVal"=w171:bool)  [unwired: 1 in, 5 out]
                n60 = case shown="True" w171 {
                  selector: w171 -> [w182 _]
                  tunnel: w175 -> [w183 w203]
                  tunnel: w174 -> [w180 w214]
                  tunnel: [w180 w233] -> w173
                  tunnel: [w177 w232] -> w172
                  tunnel: w171 -> [_ w231]
                  tunnel: [w176 Page_-_Execute_State."Idle"] -> w170
                  frame False {
                    n61 = local read "Hold Time Remainder"() -> (w179:dbl)
                    n62 = Bundle By Name(cluster=w183, "Holding Starter?"=w182) -> (w178:T13)
                    n63 = Greater Than 0?(x=w179) -> (x > 0?=w181:bool)
                    n64 = case shown="True" w181 {
                      tunnel: w178 -> [w185 w194]
                      tunnel: [w185 w192] -> w177
                      tunnel: [Page_-_Execute_State."Idle" Page_-_Execute_State."Get Next Sequence"] -> w176
                      frame False {
                      }
                      frame True {
                        w186 = "Failed" ("Test Status Ind")
                        n65 = Unbundle By Name(w194) -> ("Sequence Data"=w197:T3[], "Sequence Number"=w195:i32)
                        n66 = property on="Table Reading" class="MCListbox (strict)"() -> ("ItemNames"=w190:string[][])  [unwired: 2 in, 2 out]
                        n67 = local write "Test Status Ind"(w186) -> ()
                        n68 = Index Array(array=w197, index=w195) -> (element=w199:T3)
                        n69 = Replace Array Subset(array=w190, new element=w186, index (row)=7, index (col)=1 ("disabled index (col)")) -> (w189:string[][])
                        n70 = Bundle By Name(cluster=w199, "Seq.Status"=u32 13816530) -> (w196:T3)
                        n71 = property on="Table Reading" class="MCListbox (strict)"("ItemNames"=w189) -> ()  [unwired: 2 in, 2 out]
                        n72 = Replace Array Subset(array=w197, new element=w196, index=w195) -> (w191:T3[])
                        n73 = Bundle By Name(cluster=w194, "Sequence Data"=w191) -> (w192:T13)
                        n74 = local write "Sequence List"(w191) -> ()
                        n75 = call "Gen - Popup Single Button (Auto Close).vi"("Type"=enum16{"Error", "Info"}."Error", "Message in"="Pressure Drops Below Allowable Range before test finishes.\nMoving to next sequence", "Header"="HOLDING TIME") -> ()  [unwired: 7 in, 2 out]
                      }
                    }
                  }
                  frame True {
                    w207 = 1 ("disabled index (col)")
                    n76 = local read "Hold Time (hh:mm)"() -> (w230:string)
                    n77 = local read "Current Pressure (psi)"() -> (w206:sgl)
                    n78 = Get Date/Time In Seconds() -> (seconds since 1Jan1904=w217:timestamp)
                    n79 = call <vilib>:"Delimited String to 1D String Array.vi"("delimiter"=":", "delimited string"=w230) -> ("string array"=w228:string[])  [unwired: 9 in]
                    n80 = property on="Table Reading" class="MCListbox (strict)"(error in=w214) -> (error out=w209:errorcluster, "ItemNames"=w213:string[][])  [unwired: 1 in, 1 out]
                    n81 = Format Date/Time String(time format string (%c)="%H:%M:%S %B%d, %y", seconds (now)=w217) -> (date/time string=w210:string)  [unwired: 1 in]
                    n82 = Number To Fractional String(number=w206, precision (6)=i16 1) -> (F-format string=w204:string)  [unwired: 2 in]
                    n83 = Index Array(array=w228) -> (element #1=w227:string, element #2=w226:string)  [unwired: 2 in]
                    n84 = Decimal String To Number(string=w227) -> (number=w225:i32)  [unwired: 2 in, 1 out]
                    n85 = Decimal String To Number(string=w226) -> (number=w222:i32)  [unwired: 2 in, 1 out]
                    n86 = Replace Array Subset(array=w213, new element #1=w210, index (row) #1=0 ("disabled index (row)"), index (col) #1=w207, new element #2=w204, index (row) #2=3 ("index (row)"), index (col) #2=w207) -> (w212:string[][])
                    n87 = Multiply(x=3600, y=w225) -> (x*y=w223:i32)
                    n88 = Multiply(x=60, y=w222) -> (x*y=w220:i32)
                    n89 = property on="Table Reading" class="MCListbox (strict)"(error in=w209, "ItemNames"=w212) -> (error out=w215:errorcluster)  [unwired: 1 in, 1 out]
                    n90 = Add(x=w223, y=w220) -> (x+y=w219:i32)
                    n91 = Bundle By Name(cluster=w203, "Holding Starter?"=w231, "Remaining Holding Time"=w219, "Target Holding Time"=w219) -> (w232:T13)
                    n92 = property on="Start Mark" class="Bool (strict)"(error in=w215, "Val(Sgnl)"=w231) -> (error out=w233:errorcluster)  [unwired: 1 in, 1 out]
                  }
                }
              }
              event "TARE": Value Change {
                n93 = event-data() -> ()  [unwired: 1 in, 1 out]
                n94 = Unbundle By Name(w239) -> ("AI Offset"=w238:sgl[], "Event AI Data"=w234:sgl[])
                n95 = property on="Current Pressure (psi)" class="DigNum (strict)" props=["Value"](error in=w241) -> (error out=w240:errorcluster)  [unwired: 1 in, 2 out]
                n96 = Add(x=w238, y=w234) -> (x+y=w236:sgl[])
                n97 = Bundle By Name(cluster=w239, "AI Offset"=w236) -> (w237:T13)
              }
              event "End Mark": Value Change {
                w245 = u32 1 ("Active Cursor")
                n98 = event-data() -> ()  [unwired: 1 in, 1 out]
                n99 = Unbundle By Name(w254) -> ("Counter Time"=w243:dbl, "Point Phase"=w253:dbl[], "Current Pressure"=w242:sgl)
                n100 = Insert Into Array(array=w253, new element=w243) -> (w251:dbl[])  [unwired: 1 in]
                n101 = Bundle By Name(cluster=T16 {"X"=0.0, "Y"=0.0} ("Cursor.Cursor Position"), "Y"=w242, "X"=w243) -> (w247:T16)
                n102 = property on="Linear Graph" class="XYGraph (strict)"(error in=w250, "Active Cursor"=w245, "Cursor.Cursor Color"="Stop Marker", "Cursor.Cursor Position"=w247, "Cursor.Visible"=TRUE) -> (error out=w249:errorcluster)  [unwired: 1 in, 1 out]
                n103 = Bundle By Name(cluster=w254, "Point Phase"=w251, "marking plot colour"="Stop Marker", "Active Cursor"=w245) -> (w252:T13)
              }
              event "Clear Mark": Value Change {
                n104 = event-data() -> ()  [unwired: 1 in, 1 out]
                n105 = Unbundle By Name(w266) -> ("Point Phase"=w265:dbl[], "Active Cursor"=w258:u32)
                n106 = Reverse 1D Array(array=w265) -> (reversed array=w269:dbl[])
                n107 = Delete From Array(array=w269, length=1, index=0) -> (array with subset deleted=w256:dbl[])  [unwired: 1 out]
                n108 = property on="Linear Graph" class="XYGraph (strict)"(error in=w261, "Active Cursor"=w258, "Cursor.Visible"=FALSE) -> (error out=w260:errorcluster)  [unwired: 1 in, 1 out]
                n109 = Reverse 1D Array(array=w256) -> (reversed array=w263:dbl[])
                n110 = Bundle By Name(cluster=w266, "Point Phase"=w263, "Start Mark"=FALSE) -> (w264:T13)
              }
              event "View": Value Change {
                n111 = event-data() -> ("NewVal"=w274:string)  [unwired: 1 in]
                n112 = case shown="\"Polar Plot\", Default" w274 {
                  tunnel: w275 -> [w278 w280 w282 w283]
                  tunnel: [w278 w280 w282 w283] -> w273
                  tunnel: [T1."Polar Plot" ("tab - View Data") T1."Linear" ("tab - View Data") T1."Statistic" ("tab - View Data") T1."Key Value" ("tab - View Data")] -> w270
                  frame "Polar Plot", Default {
                  }
                  frame "Linear" {
                  }
                  frame "Statistic" {
                  }
                  frame "Key Value" {
                  }
                }
                n113 = property on="tab - View Data" class="TabCtl (strict)"(error in=w273, "Value"=w270) -> (error out=w272:errorcluster)  [unwired: 1 in, 1 out]
              }
              event "Finish": Value Change {
                n114 = event-data() -> ()  [unwired: 1 in, 6 out]
              }
              event "Stop": Value Change {
                n115 = event-data() -> ()  [unwired: 1 in, 6 out]
              }
              event User Event {
                n116 = event-data() -> ()  [unwired: 1 in, 5 out]
              }
            }
            n117 = Bundle By Name(cluster=w109, "Event Ref"=w105) -> (w106:T13)
          }
          frame "Clear Mark" {
            n118 = Unbundle By Name(w295) -> ("Point Phase"=w301:dbl[])
            n119 = Array Size(array=w301) -> (size(s)=w300:i32)
            n120 = Not Equal?(x=w300, y=1) -> (x != y?=w296:bool)
            n121 = case shown="False" w296 {
              tunnel: w298 -> [w306 w314]
              tunnel: [w305 w314] -> w297
              tunnel: w295 -> [w310 w313]
              tunnel: [w312 w313] -> w294
              frame False {
                n122 = Unbundle By Name(w310) -> ("Array of Elapse Time"=w309:timestamp[])
                n123 = Get Date/Time In Seconds() -> (seconds since 1Jan1904=w307:timestamp)
                n124 = Replace Array Subset(array=w309, new element=w307, index=Execute_-_Index_of_Elapse_time."Holding Time") -> (w311:timestamp[])
                n125 = property on="End Holding Datetime" class="Str"(error in=w306, "Value"="" ("End Holding Datetime")) -> (error out=w305:errorcluster)  [unwired: 1 in, 1 out]
                n126 = Bundle By Name(cluster=w310, "Array of Elapse Time"=w311) -> (w312:T13)
              }
              frame True {
              }
            }
          }
          frame "Start Marking" {
            n127 = Unbundle By Name(w317) -> ("Start Mark"=w316:bool)
            n128 = case shown="False" w316 {
              tunnel: [w323 w350] -> w318
              tunnel: [w322 w329] -> w319
              tunnel: [Page_-_Execute_State."Idle" Page_-_Execute_State."Idle"] -> w315
              tunnel: w320 -> [w322 w337]
              tunnel: w317 -> [w323 w336]
              frame True {
              }
              frame False {
                w346 = u32 0 ("Active Cursor")
                n129 = Unbundle By Name(w336) -> ("Array of Elapse Time"=w335:timestamp[], "Point Phase"=w332:dbl[], "Counter Time"=w328:dbl, "Current Pressure"=w325:sgl)
                n130 = Insert Into Array(array=w332, new element=w328) -> (w349:dbl[])  [unwired: 1 in]
                n131 = Bundle By Name(cluster=T16 {"X"=0.0, "Y"=0.0} ("Cursor.Cursor Position"), "Y"=w325, "X"=w328) -> (w348:T16)
                n132 = Get Date/Time In Seconds() -> (seconds since 1Jan1904=w343:timestamp)
                n133 = property on="Linear Graph" class="XYGraph (strict)"(error in=w337, "Active Cursor"=w346, "Cursor.Cursor Color"="Start Marker", "Cursor.Cursor Position"=w348, "Cursor.Visible"=TRUE) -> (error out=w330:errorcluster)  [unwired: 1 in, 1 out]
                n134 = To Long Integer(number=Execute_-_Index_of_Elapse_time."Holding Time") -> (32bit integer=w334:i32)
                n135 = Replace Array Subset(array=w335, new element=w343, index=w334) -> (w342:timestamp[])
                n136 = Get Date/Time In Seconds() -> (seconds since 1Jan1904=w339:timestamp)
                n137 = Format Date/Time String(time format string (%c)="%d.%B.%Y %H:%M:%S" ("format string"), seconds (now)=w339) -> (date/time string=→"Start Holding Datetime":string)  [unwired: 1 in]
                n138 = Format Into String(format string="%.1f", error in=w330, w325) -> (resulting string=→"Start Holding Pressure (psi)":string, error out=w329:errorcluster)  [unwired: 1 in]
                n139 = Bundle By Name(cluster=w336, "Start Mark"=TRUE, "Array of Elapse Time"=w342, "Point Phase"=w349, "marking plot colour"="Start Marker", "Active Cursor"=w346, "Start Holding Pressure (psi)"=w325) -> (w350:T13)
              }
            }
          }
          frame "Init Test Param" {
            w359 = sgl[] [] ("Magnitude ,y")
            n140 = Unbundle By Name(w367) -> ("Array of Elapse Time"=w376:timestamp[], "Config.Holding Pressure"=w357:dbl)
            n141 = property on="Recording Duration" class="Str"(error in=w363, "Value"="00:00:00" ("Recording Duration")) -> (error out=w362:errorcluster)  [unwired: 1 in, 1 out]
            n142 = Get Date/Time In Seconds() -> (seconds since 1Jan1904=w374:timestamp)
            n143 = Multiply(x=w357, y=1.25) -> (x*y=w355:dbl)
            n144 = for {
              N: 2 -> [_]
              tunnel: [w382] -> w365
              tunnel: w362 -> [w379]
              tunnel: w355 -> [w378]
              i -> [w381]
              n145 = property on="Linear Graph" class="XYGraph (strict)"(error in=w379, "Active Cursor"=w381, "Cursor.Visible"=FALSE, "YScale.Maximum"=w378) -> (error out=w382:errorcluster)  [unwired: 1 in, 1 out]
            }
            n146 = To Long Integer(number=Execute_-_Index_of_Elapse_time."Elapse Gap Data") -> (32bit integer=w375:i32)
            n147 = To Long Integer(number=Execute_-_Index_of_Elapse_time."Recording Duration") -> (32bit integer=w373:i32)
            n148 = Replace Array Subset(array=w376, new element #1=w374, index #1=w375, new element #2=w374, index #2=w373) -> (w377:timestamp[])
            n149 = Initialize Array(0.0, 3 ("dimension size")) -> (w351:dbl[])
            n150 = Bundle By Name(cluster=w367, "Array of Elapse Time"=w377, "Counter Time"=0.0 ("Counter"), "Magnitude ,y"=w359, "Time ,x"=w359, "Run Test"="Run Test", "Start Mark"=FALSE, "T_Out"=-1, "Result Elapse"=w351) -> (w366:T13)
          }
          frame "Init File and Folder" {
            w383 = "Testing" ("Test Status Ind")
            n151 = Unbundle By Name(w417) -> ("Current Sequence.Seq.No"=w395:string, "Data to Execute.Transaction Info.Transaction Number"=w416:u32)
            n152 = call "FGV - Data Path.vi"("FGV State"=State_-_FGV."Read", "Error In"=w419) -> ("Error Out"=w393:errorcluster, "Path Out"=w415:path)  [unwired: 8 in]
            n153 = Number To Decimal String(number=w416) -> (decimal integer string=w412:string)  [unwired: 1 in]
            n154 = Build Path(base path=w415, name or relative path=path "Results") -> (appended path=w413:path)
            n155 = Build Path(base path=w413, name or relative path=w412) -> (appended path=w397:path)
            n156 = Concatenate Strings("SeqNo" ("string"), w395) -> (w394:string)
            "SequenceNoFolder" <- w394
            n157 = Build Path(base path=w397, name or relative path=w394) -> (appended path=w391:path)
            n158 = Create Folder(path (use dialog)=w391, error in=w393) -> (created path=w390:path, error out=w392:errorcluster)  [unwired: 1 in, 1 out]
            n159 = Build Path(base path=w390, name or relative path=path "Data.csv") -> (appended path=w406:path)
            n160 = Unbundle By Name(w417) -> ("Sequence Data"=w402:T3[], "Sequence Number"=w400:i32)
            n161 = Index Array(array=w402, index=w400) -> (element=w404:T3)
            n162 = Bundle By Name(cluster=w404, "Seq.Status"=u32 3381759) -> (w401:T3)
            n163 = property on="Table Reading" class="MCListbox (strict)"() -> ("ItemNames"=w387:string[][])  [unwired: 2 in, 2 out]
            n164 = local write "Test Status Ind"(w383) -> ()
            n165 = Replace Array Subset(array=w402, new element=w401, index=w400) -> (w388:T3[])
            n166 = call-poly <vilib>:"Write Delimited Spreadsheet.vi"("file path (dialog if empty)"=w406, "1D data"=string[] ["Timestamp", "Pressure 1", "Pressure 2", "Pressure 3", "Pressure 4"], "append to file? (new file:F)"=FALSE, "error in (no error)"=w392, "delimiter (\\t)"="," ("delimiter (\\t)")) -> ("new file path (Not A Path if cancelled)"=w398:path, "error out"=w407:errorcluster)  [unwired: 9 in]
            n167 = Replace Array Subset(array=w387, new element=w383, index (row)=7, index (col)=1 ("disabled index (col)")) -> (w386:string[][])
            n168 = local write "Sequence List"(w388) -> ()
            n169 = property on="Table Reading" class="MCListbox (strict)"("ItemNames"=w386) -> ()  [unwired: 2 in, 2 out]
            n170 = Bundle By Name(cluster=w417, "Sequence Data"=w388, "Datalog path"=w398, "Sequence Started"=TRUE) -> (w399:T13)
          }
          frame "Get Current Sequence" {
            w435 = FALSE ("Run Test")
            n171 = Unbundle By Name(w447) -> ("Sequence Data"=w446:T3[], "Sequence Number"=w445:i32)
            n172 = Index Array(array=w446, index=w445) -> (element=w436:T3)
            n173 = Bundle By Name(cluster=w447, "Current Sequence"=w436, "Run Test"=w435, "Sequence Started"=w435) -> (w434:T13)
            n174 = Unbundle By Name(w436) -> ("Seq.TestSequence"=→"Test Sequence":string, "Seq.No"=→"Seq.No":string, "Seq.TestReq"=→"Test Requirement":string, "Seq.Variance"=→"Variance":string, "Seq.TestMedia"=→"Test Media":string, "Seq.TestPressure"=w450:string, "Seq.HoldingTime"=→"Hold Time (hh:mm)":string, "Seq.BDIndicator"=w449:string)  [unwired: 4 out]
            n175 = Decimal String To Number(string=w450) -> (number=w431:i32)  [unwired: 2 in, 1 out]
            "Test Pressure" <- w431
            n176 = Equal?(x=w449, y="Y") -> (x = y?=→"Blow Down  Test":bool)
            n177 = property on="Table Reading" class="MCListbox (strict)"() -> ("ItemNames"=w430:string[][])  [unwired: 2 in, 2 out]
            n178 = Unbundle By Name(w434) -> ("Data to Execute.Acceptance Criteria Info.Permitted Hold Pressure Drop"=w426:dbl)
            n179 = property on="Run Test" class="Bool (strict)"(error in=w422, "Val(Sgnl)"=FALSE ("Value (Signaling)")) -> (error out=w421:errorcluster)  [unwired: 1 in, 1 out]
            n180 = Divide(x=w426, y=100.0) -> (x/y=w432:dbl)
            n181 = Multiply(x=w432, y=w431) -> (x*y=w427:dbl)
            n182 = Format Into String(format string="%.1f(%d%%)", w427, w426) -> (resulting string=w423:string)  [unwired: 2 in, 1 out]
            n183 = Replace Array Subset(array=w430, new element=w423, index (row)=6, index (col)=1 ("disabled index (col)")) -> (w429:string[][])
            n184 = property on="Table Reading" class="MCListbox (strict)"("ItemNames"=w429) -> ()  [unwired: 2 in, 2 out]
          }
          frame "Cal Elapse Time" {
            n185 = Unbundle By Name(w462) -> ("Array of Elapse Time"=w468:timestamp[], "Holding Starter?"=w463:bool)
            n186 = Index Array(array=w468, index #1=Execute_-_Index_of_Elapse_time."Recording Duration", index #2=Execute_-_Index_of_Elapse_time."Holding Time", index #3=Execute_-_Index_of_Elapse_time."Elapse Gap Data") -> (element #1=w464:timestamp, element #2=w453:timestamp, element #3=w451:timestamp)
            n187 = Get Date/Time In Seconds() -> (seconds since 1Jan1904=w454:timestamp)
            n188 = Unbundle By Name(w462) -> ("Result Elapse"=w461:dbl[])
            n189 = case shown="True" w463 {
              tunnel: w454 -> [_ w477]
              tunnel: w453 -> [w474 w476]
              tunnel: [w473 w475] -> w456
              frame False {
                n190 = To Double Precision Float(number=w474) -> (double precision float=w473:dbl)
              }
              frame True {
                n191 = Subtract(x=w477, y=w476) -> (x-y=w475:dbl)
              }
            }
            n192 = Subtract(x=w454, y=w464) -> (x-y=w458:dbl)
            n193 = Subtract(x=w454, y=w451) -> (x-y=w452:dbl)
            n194 = Replace Array Subset(array=w461, new element #1=w458, index #1=Execute_-_Index_of_Elapse_time."Recording Duration", new element #2=w456, index #2=Execute_-_Index_of_Elapse_time."Holding Time", new element #3=w452, index #3=Execute_-_Index_of_Elapse_time."Elapse Gap Data") -> (w460:dbl[])
            n195 = Bundle By Name(cluster=w462, "Result Elapse"=w460) -> (w470:T13)
          }
          frame "Display Data" {
            # "Display Pressure Data and recording Duration"
            n196 = Unbundle By Name(w488) -> ("Event AI Data"=w492:sgl[], "AI Offset"=w503:sgl[], "Result Elapse"=w502:dbl[], "Run Test"=w497:bool)
            n197 = To Long Integer(number=Execute_-_Index_of_Elapse_time."Recording Duration") -> (32bit integer=w498:i32)
            n198 = Index Array(array=w502, index=w498) -> (element=w499:dbl)
            n199 = case shown="True" w497 {
              tunnel: w501 -> [w508 w512]
              tunnel: [w508 w511] -> w490
              tunnel: w499 -> [_ w510]
              frame False {
              }
              frame True {
                n200 = Format Into String(format string="%<%H:%M:%S>t", error in=w512, w510) -> (resulting string=→"Recording Duration" →"Key Value Recording Duration":string, error out=w511:errorcluster)  [unwired: 1 in]
              }
            }
            n201 = Get Date/Time In Seconds() -> (seconds since 1Jan1904=w483:timestamp)
            n202 = Unbundle By Name(w488) -> ("Datalog path"=w487:path)
            n203 = Format Date/Time String(time format string (%c)="%d/%m/%Y %H:%M:%S", seconds (now)=w483) -> (date/time string=w480:string)  [unwired: 1 in]
            n204 = Subtract(x=w492, y=w503) -> (x-y=w481:sgl[])
            n205 = for {
              tunnel: w481 -> [w507] mode=indexing
              tunnel: [w506] -> w479 mode=indexing
              n206 = Number To Fractional String(number=w507, precision (6)=i16 1) -> (F-format string=w506:string)  [unwired: 2 in]
            }
            n207 = Index Array(array=w481) -> (element=w491:sgl)  [unwired: 1 in]
            "Current Pressure (psi)" <- w491
            "Key Value Current Pressure (psi)" <- w491
            n208 = Build Array (concatenate)(w480, w479) -> (w478:string[])
            n209 = local read "Test Pressure"() -> (w495:i32)
            n210 = call "Check Pressure Stabilize.vi"("Numeric in"=w491, "Test Pressure"=w495) -> ("Numeric out"=w493:sgl)  [unwired: 9 in]
            n211 = call-poly <vilib>:"Write Delimited Spreadsheet.vi"("file path (dialog if empty)"=w487, "format (%s)"="%s" ("format (%.3f)"), "1D data"=w478, "append to file? (new file:F)"=TRUE, "error in (no error)"=w490, "delimiter (\\t)"="," ("delimiter (\\t)")) -> ("error out"=w489:errorcluster)  [unwired: 8 in, 1 out]
            n212 = local write "%Pressure Stabilized"(w493) -> ()
            n213 = Bundle By Name(cluster=w488, "Current Pressure"=w491, "%Pressure Stabilized"=w493) -> (w496:T13)
          }
          frame "Check Start Holding" {
            n214 = Unbundle By Name(w525) -> ("%Pressure Stabilized"=w524:dbl, "Data to Execute.Acceptance Criteria Info.Max Start Hold Pressure"=w521:dbl, "Data to Execute.Execution Info.Auto Set Marker"=w517:bool)
            n215 = Subtract(x=100.0, y=w524) -> (x-y=w522:dbl)
            n216 = Less Or Equal?(x=w522, y=w521) -> (x <= y?=w515:bool)
            n217 = call-poly <userlib>:"Data Changed__ogtk.vi"("Boolean"=w515) -> ("Changed"=w518:bool)
            n218 = Compound Arithmetic op=AND(TRUE ("value"), w518, w517) -> (w516:bool)
            n219 = case shown="True" w516 {
              tunnel: w520 -> [w530 w533]
              tunnel: [w530 w532] -> w519
              tunnel: w515 -> [_ w531]
              frame False {
              }
              frame True {
                n220 = property on="Holding Started" class="Bool (strict)"(error in=w533, "Val(Sgnl)"=w531) -> (error out=w532:errorcluster)  [unwired: 1 in, 1 out]
              }
            }
            n221 = Unbundle By Name(w525) -> ("Run Test"=w526:bool)
            n222 = Select(t=Page_-_Execute_State."Polar attributes", s=w526, f=Page_-_Execute_State."Idle") -> (s? t:f=w527:T14)
          }
          frame "Polar attributes" {
            w549 = 1000.0 ("y")
            # "Auto Scale"
            # "Set-up Polar attribute"
            n223 = Unbundle By Name(w544) -> ("Max Pressure"=w543:sgl, "Current Pressure"=w540:sgl)
            n224 = Greater Or Equal?(x=w543, y=w540) -> (x >= y?=w545:bool)
            n225 = Select(t=w543, s=w545, f=w540) -> (s? t:f=w539:sgl)
            n226 = Equal To 0?(x=w539) -> (x = 0?=w553:bool)
            n227 = Select(t=100.0, s=w553, f=w539) -> (s? t:f=w551:dbl)
            n228 = Multiply(x=w551, y=1.25) -> (x*y=w547:dbl)
            n229 = Divide(x=w547, y=w549) -> (x/y=w550:dbl)
            n230 = Round Toward +Infinity(x=w550) -> (ceil(x): smallest int >= x=w548:dbl)
            n231 = Multiply(x=w548, y=w549) -> (x*y=w538:dbl)
            n232 = Format Into String(format string="%.1f", w538) -> (resulting string=w536:string)  [unwired: 2 in, 1 out]
            n233 = Bundle By Name(cluster=w544, "Display Polar Scale.Max Scale label"=w536, "Max Pressure"=w539, "polar attributes.grid color"="Grid Colour", "polar attributes.plot color"="Plot Colour", "polar attributes.maximum"=w538, "polar attributes.minimum"=0.0 ("minimum"), "polar attributes.fmt and prec.format"=T18."Decimal" ("fmt and prec.format"), "Plot and scale.Size Linear plot"=u16 3, "Plot and scale.Size point plot"=u16 6) -> (w554:T13)
          }
          frame "Insert Acc Data" {
            # "Insert pressure to array of magnitude"
            n234 = Unbundle By Name(w575) -> ("Magnitude ,y"=w574:sgl[], "Current Pressure"=w573:sgl, "Time ,x"=w572:dbl[], "Result Elapse"=w571:dbl[], "Counter Time"=w569:dbl)
            n235 = To Long Integer(number=Execute_-_Index_of_Elapse_time."Elapse Gap Data") -> (32bit integer=w560:i32)
            n236 = Index Array(array=w571, index=w560) -> (element=w570:dbl)
            n237 = Add(x=w570, y=w569) -> (x+y=w565:dbl)
            n238 = Insert Into Array(array=w572, new element=w569) -> (w566:dbl[])  [unwired: 1 in]
            n239 = Insert Into Array(array=w574, new element=w573) -> (w567:sgl[])  [unwired: 1 in]
            n240 = Bundle By Name(cluster=w575, "Magnitude ,y"=w567, "Time ,x"=w566, "Counter Time"=w565) -> (w568:T13)
          }
          frame "Convert Time To Phase" {
            # "Convert time to phase"
            n241 = Unbundle By Name(w590) -> ("Magnitude ,y"=w583:sgl[], "Time ,x"=w589:dbl[], "Plot length scale"=w577:dbl, "Point Phase"=w579:dbl[])
            n242 = Multiply(x=w589, y=w577) -> (x*y=w584:dbl[])
            n243 = for {
              shift-right: [w597] -> w585
              shift-left: w586 -> [w597]
              tunnel: w584 -> [w592] mode=indexing
              tunnel: w583 -> [w594] mode=indexing
              tunnel: [w595] -> w580 mode=indexing
              tunnel: [w592] -> w581
              tunnel: w577 -> [w591]
              tunnel: [w591] -> w576
              n244 = To Double Precision Float(number=w594) -> (double precision float=w593:dbl)
              n245 = Bundle By Name(cluster=cluster{"magnitude":dbl, "phase":dbl} {"magnitude"=0.0, "phase"=0.0} ("data array [mag, phase (deg)]"), "magnitude"=w593, "phase"=w592) -> (w595:cluster{"magnitude":dbl, "phase":dbl})
            }
            n246 = call "Execute Search To Mark.vi"("Plot length scale"=w576, "Point Phase"=w579, "Data [magnitude,Phase]In"=w580) -> ("Data [magnitude,Phase] Out"=w578:cluster{"magnitude 2":dbl, "phase":dbl}[])  [unwired: 8 in]
            n247 = Bundle By Name(cluster=w590, "data array [mag, phase (deg)]"=w580, "Max Phase"=w581, "Marking Data"=w578) -> (w587:T13)
          }
          frame "Get Plot length" {
            n248 = Unbundle By Name(w616) -> ("Plot length (min)"=w615:dbl, "Plot length scale"=w614:dbl, "Max Phase"=w613:dbl)
            n249 = call "Get plot length.vi"("Max phase"=w613, "Plot length scale"=w614, "Plot length (min)"=w615) -> ("New plot length scale"=w611:dbl, "New plot length"=w600:dbl)
            n250 = Multiply(x=w600, y=60.0) -> (x*y=w606:dbl)
            n251 = To Long Integer(number=w600) -> (32bit integer=w608:i32)
            n252 = Multiply(x=w606, y=dbl[] [0.0, 0.041666666666666664, 0.08333333333333333, 0.125, 0.16666666666666666, 0.20833333333333334, 0.25, 0.2916666666666667, 0.3333333333333333, 0.375, 0.4166666666666667, 0.4583333333333333, 0.5, 0.5416666666666666, 0.5833333333333334, 0.625, 0.6666666666666666, 0.7083333333333334, 0.75, 0.7916666666666666, 0.8333333333333334, 0.875, 0.9166666666666666, 0.9583333333333334, 1.0] ("Array 2")) -> (x*y=w605:dbl[])
            n253 = Format Into String(format string="%d", w608) -> (resulting string=w607:string)  [unwired: 2 in, 1 out]
            n254 = for {
              tunnel: w605 -> [w620] mode=indexing
              tunnel: [w618] -> w599 mode=indexing
              shift-right: [w617] -> w601
              shift-left: w602 -> [w617]
              n255 = Number To Fractional String(number=w620, precision (6)=i16 1) -> (F-format string=w618:string)  [unwired: 2 in]
            }
            n256 = Bundle By Name(cluster=w616, "Display Polar Scale.Time Scale Label"=w607, "Plot length (min)"=w600, "Plot length scale"=w611, "axis labels"=w599) -> (w612:T13)
          }
          frame "Polar linear Plot" {
            # "plot polar data"
            n257 = Unbundle By Name(w631) -> ("Display Polar Scale"=w625:T24, "Plot and scale"=w626:T25, "marking plot colour"=w627:u32, "data array [mag, phase (deg)]"=w628:cluster{"magnitude":dbl, "phase":dbl}[], "polar attributes"=w630:T26, "axis labels"=w623:string[])
            n258 = disable-structure shown="Enabled" {
              disable-tunnel: w630 -> [w643 w648]
              disable-tunnel: w629 -> [w640 w655]
              disable-tunnel: w628 -> [w639 w647]
              disable-tunnel: w627 -> [w638 _]
              disable-tunnel: w626 -> [w637 w650]
              disable-tunnel: _ -> [w636 _]
              disable-tunnel: w625 -> [w635 _]
              disable-tunnel: [w634 w656] -> w624
              disable-tunnel: w623 -> [_ w645]
              disable-tunnel: [_ w644] -> w621
              frame Disabled {
                n259 = property on="Polar Plot" class="Pict"(error in=w640) -> (error out=w642:errorcluster, "Draw Area Size"=w641:T27)  [unwired: 1 in, 1 out]
                n260 = call "Execute -Polar Plot.vi"("Marking Data"=w636, "Display Pic Parameter"=w635, "polar attributes"=w643, "Plot and scale"=w637, "error in (no error)"=w642, "Draw Area Size"=w641, "data array [mag, phase (deg)]"=w639, "Marking color"=w638) -> ("error out"=w634:errorcluster)  [unwired: 2 in, 1 out]
              }
              frame Enabled {
                n261 = Unbundle By Name(w650) -> ("Plot Scale"=w646:dbl, "Size Linear plot"=w649:u16)
                n262 = property on="Polar Plot" class="Pict"(error in=w655) -> (error out=w654:errorcluster, "Draw Area Size"=w653:T27)  [unwired: 1 in, 1 out]
                n263 = Bundle By Name(cluster=T19 {"polar attributes"={"maximum"=0.0, "minimum"=0.0, "clip to min"=FALSE, "log?(F)"=FALSE, "grid color"=6710886, "plot color"=16711680, "fmt and prec"={"format"=enum."Decimal", "precision"=0}, "visible section"=8}, "data array [mag, phase (deg)]"=[], "font"={"desired font(Application) "=enum."Application Font", "[user-specified font] "={"Font Name:"="", "Size"=0, "Strikeout?"=FALSE, "Italic?"=FALSE, "Underline?"=FALSE, "Outline?"=FALSE, "Shadow?"=FALSE, "Bold?"=FALSE}}, "Scale Polar plot"=0.2, "Size"=1} ("Polar Properties"), "Scale Polar plot"=w646, "Size"=w649, "data array [mag, phase (deg)]"=w647, "polar attributes"=w648) -> (w652:T19)
                n264 = call "Polar Plot-Linear.vi"("axis labels"=w645, "error in"=w654, "dimensions (w,h)"=w653, "Polar Properties"=w652) -> ("error Out"=w656:errorcluster, "picture out"=w644:picture)  [unwired: 6 in]
              }
            }
            n265 = Bundle By Name(cluster=w631, "Polar Picture"=w621) -> (w622:T13)
          }
          frame "Polar Point" {
            # "plot polar data"
            n266 = Unbundle By Name(w661) -> ("Polar Picture"=w658:picture, "Plot and scale"=w671:T25, "marking plot colour"=w672:u32, "Marking Data"=w673:cluster{"magnitude 2":dbl, "phase":dbl}[], "polar attributes"=w675:T26, "axis labels"=w670:string[])
            n267 = Bundle By Name(cluster=w675, "plot color"=w672) -> (w662:T26)
            n268 = Unbundle By Name(w671) -> ("Plot Scale"=w664:dbl, "Size point plot"=w665:u16)
            n269 = property on="Polar Plot" class="Pict"(error in=w674) -> (error out=w669:errorcluster, "Draw Area Size"=w668:T27)  [unwired: 1 in, 1 out]
            n270 = Bundle By Name(cluster=T19 {"polar attributes"={"maximum"=0.0, "minimum"=0.0, "clip to min"=FALSE, "log?(F)"=FALSE, "grid color"=6710886, "plot color"=16711680, "fmt and prec"={"format"=enum."Decimal", "precision"=0}, "visible section"=8}, "data array [mag, phase (deg)]"=[], "font"={"desired font(Application) "=enum."Application Font", "[user-specified font] "={"Font Name:"="", "Size"=0, "Strikeout?"=FALSE, "Italic?"=FALSE, "Underline?"=FALSE, "Outline?"=FALSE, "Shadow?"=FALSE, "Bold?"=FALSE}}, "Scale Polar plot"=0.2, "Size"=1} ("Polar Properties"), "Scale Polar plot"=w664, "Size"=w665, "data array [mag, phase (deg)]"=w673, "polar attributes"=w662) -> (w667:T19)
            n271 = call "Polar Plot-Point.vi"("axis labels"=w670, "error in"=w669, "dimensions (w,h)"=w668, "Polar Properties"=w667, "picture In"=w658) -> ("error Out"=w663:errorcluster, "picture out"=w657:picture)  [unwired: 5 in]
            n272 = Bundle By Name(cluster=w661, "Polar Picture"=w657) -> (w659:T13)
          }
          frame "Display Label" {
            n273 = Unbundle By Name(w681) -> ("Display Polar Scale.Max Scale label"=w679:string, "Display Polar Scale.Time Scale Label"=w680:string, "Polar Picture"=w678:picture)
            n274 = call <vilib>:"Space Constant.vi"() -> ("String"=w689:string)
            n275 = Concatenate Strings("1 rev = " ("text"), w680, w689, "Minute" ("string")) -> (w691:string)
            n276 = call <vilib>:"Space Constant.vi"() -> ("String"=w685:string)
            n277 = Concatenate Strings("Max Scale  = " ("text"), w679, w685, "psi" ("string")) -> (w682:string)
            n278 = call <vilib>:"Draw Text at Point.vi"("text"=w691, "origin"=cluster{"x":i16, "y":i16} {"x"=722, "y"=35}, "picture"=w678) -> ("new picture"=w687:picture)  [unwired: 7 in, 1 out]
            n279 = call <vilib>:"Draw Text at Point.vi"("text"=w682, "origin"=cluster{"x":i16, "y":i16} {"x"=722, "y"=15}, "picture"=w687) -> ("new picture"=→"Polar Plot":picture)  [unwired: 7 in, 1 out]
          }
          frame "Plot linear Graph" {
            # "Display sensor ata on linear graph"
            n280 = Unbundle By Name(w703) -> ("Array of Elapse Time"=w708:timestamp[], "Time ,x"=w711:dbl[], "Magnitude ,y"=w710:sgl[])
            n281 = Bundle By Name(cluster=cluster{"Time ,x":dbl[], "Magnitude ,y":sgl[]} {"Time ,x"=[], "Magnitude ,y"=[]}, "Time ,x"=w711, "Magnitude ,y"=w710) -> (→"Linear Graph":cluster{"Time ,x":dbl[], "Magnitude ,y":sgl[]})
            n282 = To Long Integer(number=Execute_-_Index_of_Elapse_time."Elapse Gap Data") -> (32bit integer=w705:i32)
            n283 = Get Date/Time In Seconds() -> (seconds since 1Jan1904=w704:timestamp)
            n284 = Replace Array Subset(array=w708, new element=w704, index=w705) -> (w707:timestamp[])
            n285 = Unbundle By Name(w703) -> ("Point Phase"=w702:dbl[])
            n286 = Bundle By Name(cluster=w703, "Array of Elapse Time"=w707) -> (w709:T13)
            n287 = Array Size(array=w702) -> (size(s)=w701:i32)
            n288 = Not Equal?(x=w701, y=1) -> (x != y?=w699:bool)
            n289 = Select(t=Page_-_Execute_State."Idle", s=w699, f=Page_-_Execute_State."Update Table Data") -> (s? t:f=w697:T14)
          }
          frame "Update Table Data" {
          }
          frame "Display Holding Time" {
            n290 = Unbundle By Name(w735) -> ("Result Elapse"=w733:dbl[], "Remaining Holding Time"=w728:dbl, "Target Holding Time"=w726:dbl)
            n291 = To Long Integer(number=Execute_-_Index_of_Elapse_time."Holding Time") -> (32bit integer=w731:i32)
            n292 = Index Array(array=w733, index=w731) -> (element=w730:dbl)
            n293 = Subtract(x=w728, y=w730) -> (x-y=w720:dbl)
            "Hold Time Remainder" <- w720
            n294 = Subtract(x=w726, y=w720) -> (x-y=w727:dbl)
            n295 = Divide(x=w727, y=w726) -> (x/y=w725:dbl)
            n296 = Less Than 0?(x=w720) -> (x < 0?=w722:bool)
            n297 = Multiply(x=w725, y=100.0) -> (x*y=→"% Test Completed":dbl)
            n298 = Select(t=0.0, s=w722, f=w720) -> (s? t:f=w719:dbl)
            n299 = Format Into String(format string="%<%H:%M:%S>t", error in=w740, w719) -> (resulting string=→"Remain Hold Time":string, error out=w739:errorcluster)  [unwired: 1 in]
            n300 = Less Or Equal To 0?(x=w720) -> (x <= 0?=w737:bool)
            n301 = case shown="False" w737 {
              tunnel: w739 -> [w745 w756]
              tunnel: [w745 w747] -> w738
              tunnel: w735 -> [w744 w761]
              tunnel: [w744 w760] -> w734
              tunnel: [Page_-_Execute_State."Idle" Page_-_Execute_State."Idle"] -> w729
              frame False {
              }
              frame True {
                n302 = property on="End Mark" class="Bool (strict)"(error in=w756, "Val(Sgnl)"=TRUE) -> (error out=w763:errorcluster)  [unwired: 1 in, 1 out]
                n303 = property on="End Mark" class="Bool (strict)"(error in=w763, "Value"=FALSE ("End Mark")) -> (error out=w755:errorcluster)  [unwired: 1 in, 1 out]
                n304 = property on="Run Test" class="Bool (strict)"(error in=w755, "Val(Sgnl)"=FALSE ("Value (Signaling)")) -> (error out=w746:errorcluster)  [unwired: 1 in, 1 out]
                n305 = Get Date/Time In Seconds() -> (seconds since 1Jan1904=w751:timestamp)
                n306 = property on="Table Reading" class="MCListbox (strict)"(error in=w746) -> ("ItemNames"=w752:string[][])  [unwired: 1 in, 2 out]
                n307 = Format Date/Time String(time format string (%c)="%H:%M:%S %B%d, %y", seconds (now)=w751) -> (date/time string=w754:string)  [unwired: 1 in]
                n308 = Bundle By Name(cluster=w761, "Start Mark"=FALSE) -> (w760:T13)
                n309 = Replace Array Subset(array=w752, new element=w754, index (row)=1 ("disabled index (row)"), index (col)=1 ("disabled index (col)")) -> (w753:string[][])
                n310 = property on="Table Reading" class="MCListbox (strict)"("ItemNames"=w753) -> (error out=w747:errorcluster)  [unwired: 2 in, 1 out]
              }
            }
          }
          frame "Display Result Test" {
            w766 = 1 ("index (row)")
            n311 = Unbundle By Name(w780) -> ("Start Holding Pressure (psi)"=w774:dbl, "Remaining Holding Time"=w779:dbl)
            n312 = Get Date/Time In Seconds() -> (seconds since 1Jan1904=w794:timestamp)
            n313 = Format Into String(format string="%<%H:%M:%S>t", error in=w791, w779) -> (resulting string=w765:string, error out=w775:errorcluster)  [unwired: 1 in]
            "Recorded Holding Time" <- w765
            n314 = Format Date/Time String(time format string (%c)="%H:%M:%S %B%d, %y" ("format string"), seconds (now)=w794) -> (date/time string=w773:string)  [unwired: 1 in]
            "End Holding Datetime" <- w773
            n315 = property on="Current Pressure (psi)" class="DigNum (strict)"(error in=w775) -> (error out=w790:errorcluster, "Value"=w770:sgl)  [unwired: 1 in, 1 out]
            n316 = Subtract(x=w770, y=w774) -> (x-y=w783:dbl)
            n317 = Absolute Value(x=w783) -> (abs(x)=w781:dbl)
            n318 = Format Into String(format string="%.1f", error in=w790, w770) -> (resulting string=w771:string, error out=w789:errorcluster)  [unwired: 1 in]
            "End Holding Pressure (psi)" <- w771
            n319 = Divide(x=w781, y=w774) -> (x/y=w786:dbl)
            n320 = Multiply(x=w786, y=100.0) -> (x*y=w782:dbl)
            n321 = Format Into String(format string="%.1f psi(%.1f %%)", w781, w782) -> (resulting string=w768:string)  [unwired: 2 in, 1 out]
            "Different in Holding Pressure,psi(%)" <- w768
            n322 = property on="Table Reading" class="MCListbox (strict)"(error in=w775) -> (error out=w778:errorcluster, "ItemNames"=w776:string[][])  [unwired: 1 in, 1 out]
            n323 = Replace Array Subset(array=w776, new element #1=w773, index (row) #1=w766, index (col) #1=w766, new element #2=w771, index (row) #2=4 ("index (row)"), index (col) #2=w766, new element #3=w768, index (row) #3=5 ("index (row)"), index (col) #3=w766, new element #4=w765, index (row) #4=2 ("index (row)"), index (col) #4=w766) -> (w777:string[][])
            n324 = property on="Table Reading" class="MCListbox (strict)"(error in=w778, "ItemNames"=w777) -> ()  [unwired: 1 in, 2 out]
          }
          frame "Finish Test" {
            w805 = "Passed" ("Test Status Ind")
            n325 = Unbundle By Name(w811) -> ("Sequence Data"=w814:T3[], "Sequence Number"=w812:i32)
            n326 = Index Array(array=w814, index=w812) -> (element=w816:T3)
            n327 = Bundle By Name(cluster=w816, "Seq.Status"=u32 6618880) -> (w813:T3)
            n328 = Replace Array Subset(array=w814, new element=w813, index=w812) -> (w809:T3[])
            n329 = local write "Sequence List"(w809) -> ()
            n330 = Bundle By Name(cluster=w811, "Sequence Data"=w809) -> (w810:T13)
            n331 = property on="Table Reading" class="MCListbox (strict)"() -> ("ItemNames"=w808:string[][])  [unwired: 2 in, 2 out]
            n332 = local read "SequenceNoFolder"() -> (w796:string)
            n333 = local write "Test Status Ind"(w805) -> ()
            n334 = Replace Array Subset(array=w808, new element=w805, index (row)=7, index (col)=1 ("disabled index (col)")) -> (w799:string[][])
            n335 = property on="Table Reading" class="MCListbox (strict)"("ItemNames"=w799) -> ()  [unwired: 2 in, 2 out]
            n336 = Index Array(array=w799, index (col)=1 ("disabled index (col)")) -> (element=w797:string[])  [unwired: 1 in]
            n337 = Bundle By Name(cluster=T20 {"Execute Data"=[], "Sequence no"=""} ("Data To Report"), "Execute Data"=w797, "Sequence no"=w796) -> (w801:T20)
            n338 = call "eFGV - Data to Report.vi"("Action"=State_-_eFGV."Write", "Error In"=w804, "Data To Report"=w801) -> ("Error Out"=w803:errorcluster)  [unwired: 7 in, 1 out]
          }
          frame "Save  Data" {
            n339 = Unbundle By Name(w825) -> ("Data to Execute.Transaction Info.Transaction Number"=w826:u32)
            n340 = call "FGV - Data Path.vi"("FGV State"=State_-_FGV."Read", "Error In"=w835) -> ("Error Out"=w829:errorcluster, "Path Out"=w839:path)  [unwired: 8 in]
            n341 = Build Path(base path=w839, name or relative path=path "Results") -> (appended path=w823:path)
            n342 = Number To Decimal String(number=w826) -> (decimal integer string=w824:string)  [unwired: 1 in]
            n343 = Build Path(base path=w823, name or relative path=w824) -> (appended path=w821:path)
            n344 = local read "SequenceNoFolder"() -> (w820:string)
            n345 = Build Path(base path=w821, name or relative path=w820) -> (appended path=w819:path)
            n346 = invoke on="Polar Plot" class="Pict" method="Get Image"(error in=w829) -> (error out=w828:errorcluster, "image data"=w827:T28)  [unwired: 5 in, 4 out]
            n347 = Concatenate Strings("Polar" ("string"), ".jpeg") -> (w831:string)
            n348 = Build Path(base path=w819, name or relative path=w831) -> (appended path=w833:path)
            n349 = call <vilib>:"Write JPEG File.vi"("quality (80)"=100, "error in (no error)"=w828, "image data"=w827, "path to JPEG file"=w833) -> ("error out"=w834:errorcluster)  [unwired: 6 in, 1 out]
          }
          frame "Get Next Sequence" {
            n350 = Unbundle By Name(w848) -> ("Sequence Number"=w844:i32, "Sequence Data"=w845:T3[])
            n351 = Array Size(array=w845) -> (size(s)=w843:i32)
            n352 = Decrement(x=w843) -> (x-1=w842:i32)
            n353 = Less?(x=w844, y=w842) -> (x < y?=w841:bool)
            n354 = case shown="True" w841 {
              tunnel: w848 -> [w856 w862]
              tunnel: [Page_-_Execute_State."Idle" Page_-_Execute_State."Get Current Sequence"] -> w847
              tunnel: [w855 w860] -> w846
              tunnel: w844 -> [_ w858]
              frame False {
                n355 = Bundle By Name(cluster=w856, "Sequence Number"=0, "All Sequence Done"=TRUE) -> (w855:T13)
                n356 = call "Gen - Popup Single Button (Auto Close).vi"("Message in"="All test sequence are done", "Header"="TEST SEQUENCE") -> ()  [unwired: 8 in, 2 out]
              }
              frame True {
                n357 = Increment(x=w858) -> (x+1=w859:i32)
                n358 = Bundle By Name(cluster=w862, "Sequence Number"=w859, "Sequence Started"=FALSE) -> (w860:T13)
              }
            }
          }
          frame "Create Report" {
            n359 = call <vilib>:"Create Report.vi"("report type"=Report_Type."Excel", "error in (no error)"=w867) -> ("report out"=w864:refnum<class "NI_report.lvclass">, "error out"=w866:errorcluster)  [unwired: 12 in]
            n360 = Bundle By Name(cluster=w870, "report out"=w864) -> (w865:T13)
          }
          frame "Fillup Report" {
            n361 = Unbundle By Name(w877) -> ("report out"=w876:refnum<class "NI_report.lvclass">)
            n362 = call-poly <vilib>:"Append Report Text.vi"("report in"=w876, "MS Office parameters"=T23 {"position (excel)"={"row"=0, "column"=0}, "name (excel)"="", "bookmark (word)"=""}, "text"="", "error in (no error)"=w878) -> ("report out"=w875:refnum<class "NI_report.lvclass">, "error out"=w874:errorcluster)  [unwired: 8 in, 2 out]
            n363 = call-dynamic "Dispose Report.vi"("report in"=w875, "error in (no error)"=w874) -> ("error out"=w873:errorcluster)  [unwired: 13 in]
          }
          frame "Process" {
          }
          frame "Update Info - Transaction" {
            n364 = Unbundle By Name(w902) -> ("Data to Execute.Transaction Info"=w901:T8)
            n365 = Unbundle By Name(w901) -> ("Transaction Number"=w900:u32, "Order Number"=w898:u32, "Quantity"=w899:u16, "Customer"=w896:u32, "Customer Description"=w894:string, "Project"=w893:string, "Sales Order"=w892:u32, "Material"=w890:u32, "Material Description"=w888:string, "Rework"=w887:bool, "NCR No."=w886:string, "Ref Order No."=w885:dbl, "BOM Rev."=w884:dbl)
            n366 = Number To Decimal String(number=w898) -> (decimal integer string=w897:string)  [unwired: 1 in]
            n367 = Number To Decimal String(number=w896) -> (decimal integer string=w895:string)  [unwired: 1 in]
            n368 = Number To Decimal String(number=w892) -> (decimal integer string=w891:string)  [unwired: 1 in]
            n369 = Number To Decimal String(number=w890) -> (decimal integer string=w889:string)  [unwired: 1 in]
            n370 = local write "Transaction Number"(w900) -> ()
            n371 = local write "Order Number"(w897) -> ()
            n372 = local write "Quantity"(w899) -> ()
            n373 = local write "Customer"(w895) -> ()
            n374 = local write "Customer Description"(w894) -> ()
            n375 = local write "Project"(w893) -> ()
            n376 = local write "Sale Order"(w891) -> ()
            n377 = local write "Material"(w889) -> ()
            n378 = local write "Material Description"(w888) -> ()
            n379 = local write "Rework"(w887) -> ()
            n380 = local write "NCR No."(w886) -> ()
            n381 = local write "Ref Order No."(w885) -> ()
            n382 = local write "BOM Rev."(w884) -> ()
          }
          frame "Update Info - Product" {
            n383 = Unbundle By Name(w913) -> ("Data to Execute.Product Info.Product Category"=w912:string, "Data to Execute.Product Info.Procedure No./Ref."=w911:string, "Data to Execute.Product Info.Test System"=w905:string, "Data to Execute.Product Info.Test System Description"=w910:string, "Data to Execute.Product Info.Working Pressure"=w909:string, "Data to Execute.Product Info.Rev."=w908:string, "Data to Execute.Product Info.PSL"=w907:string)
            n384 = local write "Product Category"(w912) -> ()
            n385 = local write "Procedure No./Ref."(w911) -> ()
            n386 = local write "Test System"(w905) -> ()
            n387 = local write "Test System Description"(w910) -> ()
            n388 = local write "Working Pressure"(w909) -> ()
            n389 = local write "Rev."(w908) -> ()
            n390 = local write "PSL"(w907) -> ()
            n391 = local write "Test System"(w905) -> ()
          }
          frame "Update Info - Additional Refs" {
            n392 = Unbundle By Name(w919) -> ("Data to Execute.Misc - Additional Refs"=w916:string[][])
            n393 = property on="Table.Procedure No./Ref." class="MCListbox (strict)"(error in=w918, "ItemNames"=w916) -> (error out=w917:errorcluster)  [unwired: 1 in, 1 out]
          }
          frame "Update Info - Sensors" {
            n394 = Unbundle By Name(w924) -> ("Data to Execute.Misc - Sensors"=w921:string[][])
            n395 = property on="Table.Sensor" class="MCListbox (strict)"(error in=w923, "ItemNames"=w921) -> (error out=w922:errorcluster)  [unwired: 1 in, 1 out]
          }
          frame "Update Info - Tools" {
            n396 = Unbundle By Name(w929) -> ("Data to Execute.Misc - Tools"=w926:string[][])
            n397 = property on="Table.Tool" class="MCListbox (strict)"(error in=w928, "ItemNames"=w926) -> (error out=w927:errorcluster)  [unwired: 1 in, 1 out]
          }
          frame "Update Info - Acceptance Criteria" {
            n398 = Unbundle By Name(w941) -> ("Data to Execute.Acceptance Criteria Info.Max Start Hold Pressure"=w938:dbl, "Data to Execute.Acceptance Criteria Info.Permitted Hold Pressure Drop"=w937:dbl, "Data to Execute.Acceptance Criteria Info.Enum.Max Start Hold Pressure"=w940:enum16{"%", "psi"}, "Data to Execute.Acceptance Criteria Info.Enum.Permitted Hold Pressure Drop"=w939:enum16{"%", "psi"})
            n399 = Format Into String(w940) -> (resulting string=w936:string)  [unwired: 3 in, 1 out]
            n400 = Format Into String(w939) -> (resulting string=w933:string)  [unwired: 3 in, 1 out]
            n401 = local write "Max Start Holding Pressure"(w938) -> ()
            n402 = local write "Permitted Holding Pressure Drop"(w937) -> ()
            n403 = Concatenate Strings(w936, " on top of the test pressure" ("string")) -> (w932:string)
            n404 = Concatenate Strings(w933, " per hour (vs. start holding pressure)" ("string")) -> (w931:string)
            n405 = local write "% Test Pressure"(w932) -> ()
            n406 = local write "% Permitted Holding Pressure"(w931) -> ()
          }
          frame "Update Info - Execution" {
            n407 = Unbundle By Name(w946) -> ("Data to Execute.Execution Info.Auto Set Marker"=w945:bool, "Data to Execute.Execution Info.Auto Stop Test"=w944:bool)
            n408 = local write "Auto Set Marker"(w945) -> ()
            n409 = local write "Auto Stop Test"(w944) -> ()
          }
          frame "Update Info - Results" {
            n410 = Unbundle By Name(w951) -> ("Data to Execute.Results Info.ListBox.Output Set"=w950:string, "Data to Execute.Results Info.Output Set Description"=w949:string)
            n411 = local write "ListBox.Output Set"(w950) -> ()
            n412 = local write "Output Set Company"(w949) -> ()
          }
          frame "Update Info - Notes" {
            n413 = Unbundle By Name(w954) -> ("Data to Execute.Notes"=w953:string)
            n414 = local write "Notes"(w953) -> ()
          }
          frame "Close" {
            n415 = Unbundle By Name(w958) -> ("Event Ref"=w957:refnum<event-registration>)
            n416 = Unregister For Events(event registration refnum=w957, error in=w962) -> (error out=w961:errorcluster)
          }
        }
      }
      frame Error {
        n417 = call <vilib>:"Clear Errors.vi"("error in (no error)"=w966) -> ("error out"=w969:errorcluster)  [unwired: 5 in, 1 out]
        n418 = call "Gen - Get Application Kind.vi"("Error In"=w969) -> ("Error Out"=w965:errorcluster, "Application:Kind"=w968:T29)  [unwired: 9 in]
        n419 = Format Into String(error in=w965, w963) -> (resulting string=w964:string)  [unwired: 2 in, 1 out]
        n420 = case shown="\"Development System\"" w968 {
          tunnel: [w973 w978 w982] -> w967
          tunnel: w966 -> [w973 w975 w980]
          tunnel: w964 -> [_ w974 _]
          frame "invalid app kind", Default {
          }
          frame "Run Time System" {
            n421 = control-ref of="This VI"() -> (w976:refnum<vi>)
            n422 = call "eFGV - Generated Error.vi"("eFGV States"=State_-_eFGV."Write", "Error In"=w975, "State"=w974, "This VI"=w976) -> ("Error Out"=w978:errorcluster)  [unwired: 6 in, 1 out]
          }
          frame "Development System" {
            n423 = call <vilib>:"Simple Error Handler.vi"("error in (no error)"=w980) -> ("error?"=w979:bool, "error out"=w981:errorcluster)  [unwired: 4 in, 3 out]
            n424 = case shown="False" w979 {
              tunnel: [w983 w985] -> w982
              tunnel: w981 -> [w983 w984]
              frame False {
              }
              frame True {
                n425 = call <vilib>:"Clear Errors.vi"("error in (no error)"=w984) -> ("error out"=w985:errorcluster)  [unwired: 5 in, 1 out]
              }
            }
          }
        }
      }
    }
  }
  n426 = disable-structure shown="Disabled" {
    frame Disabled {
      n427 = call "eFGV - Data to Report.vi"() -> ("Error Out"=w988:errorcluster, "Data To Report"=w986:refnum<user-event>, "Action"=w987:T21)  [unwired: 9 in]
    }
    frame Enabled {
    }
  }
